vi "Pick&Place_module.vi"() -> ()   [LabVIEW 2016]
uses:
  Classes/Controllers/I-O/Copy of NI-DAQ Folder/NI-DAQ.lvclass
  D:/INTT/V1/Classes/Controllers/I-O/Copy of I-O Folder/I-O.lvclass
  Classes/Controllers/Dispenser/Copy of Ultimus V2 Folder/Ultimus V2.lvclass
  <vilib>/Analysis/coordinate.llb/2D Cartesian Coordinate Rotation (Scalar).vi
  <vilib>/Utility/file.llb/Read Delimited Spreadsheet (DBL).vi
  <vilib>/Utility/file.llb/Write Delimited Spreadsheet (DBL).vi
  Classes/Controllers/Motion/Copy of Motion Folder/Motion.lvclass
  Classes/Controllers/Camera/Copy of Controller Folder/Controller.lvclass
  <vilib>/Analysis/NI_AALPro.lvlib
  Classes/Controllers/I-O/Copy of I-O Folder/I-O.lvclass
panel:
  in  "Ultimus Pressure":i16=20
  in  "Values":bool[](array[boolean])=[FALSE, FALSE]
  out "vacuum on?":bool[](array[boolean])
  out "Array 2":dbl[][](array[numeric])
  out "Measured PickupTool position":dbl[][](array[numeric])
  in  "sampel vacuum":i32[](array[numeric])=[15, 19]
  in  "VacChannel for sample":i32=1
  in  "TrayVaccum":bool
  in  "check height? 2":bool
  in  "check height?":bool
  out "Needle parking position":dbl[](array[numeric])
  out "GlueBox":dbl[][](array[numeric])
  out "appended array":dbl[][](array[numeric])
  in  "chip placement height compensation":dbl=-0.47 format="%#_13g"
  out "Sample on HDI":dbl[][](array[numeric]) format="%#_8g"
  in  "Sensor A/B":bool
  out "Gantry current position":dbl[](array[numeric])
  in  "READ Position":bool
  in  "Needle Height Compenstation\n(glue gap)":dbl=0.34
  in  "Needle Alignment":bool
  in  "Parking position":dbl[](array[numeric])=[625.0, 625.0, 0.0, 0.01]
  in  "GOTO":bool
  in  "Default Pickup Tool Position":dbl[][](array[numeric])=[[153.043, 779.997, 54.962, 0.0365632], [153.043, 779.997, 54.962, 0.0365632]]
  in  "Number of Chips/Sensors \nto be assembled":i32=1
  in  "Default HDI alignment \nmark position":dbl[](array[numeric])=[292.437, 991.477, 79.3487, -0.011805]
  in  "Default HDI size":dbl[](array[numeric])=[24.3371, 231.337, -0.0132064, -0.000194865]
  out "# of tasks excuted":i32
  out "Chips on tray position":dbl[][](array[numeric])
  out "measured HDI size":dbl[](array[numeric])
  in  "Chip tray":dbl[](array[numeric])=[465.031, 710.639, 69.8028, 0.00407755]
  out "Sample position \non HDI":dbl[][](array[numeric])
  in  "Inititalize":bool
  in  "Pick and place":bool
  in  "Deposit Glue":bool
  in  "Measure Pickup Tools":bool
  in  "Measure Samples on tray":bool
  out "default chip and sensor position w.r.t. 1st mark":dbl[][](array[numeric])
  in  "Assembly Type":bool=TRUE
  in  "Stop":bool
  in  "Measure HDI":bool
  out "Measure HDI top-left":dbl[](array[numeric])
  # "Sensor Tray \nVacuum Channel"
  # "Chips"
  # "Sensor 0.3 -> 200 micron glue thickness\nChips 0.34-> 150 micron glue thickness"
  # "Sensors"
  # "Sensor B short"
  # "Sensors B\n(Short)"
  # "Sensors A\n(Long)"
  # "Chips : -0.47-> 60 micron height gap\n               -0.5 -> 90 micron"
  # "Sensor A long"
  # "ACTIONS"
  # "HDI infomation"
  # "chips use channel 0, 2\nsensors use channel 0, 1"
  # "sensor height 69.8471\nchip height 84.693"
  # "Pick and Place"
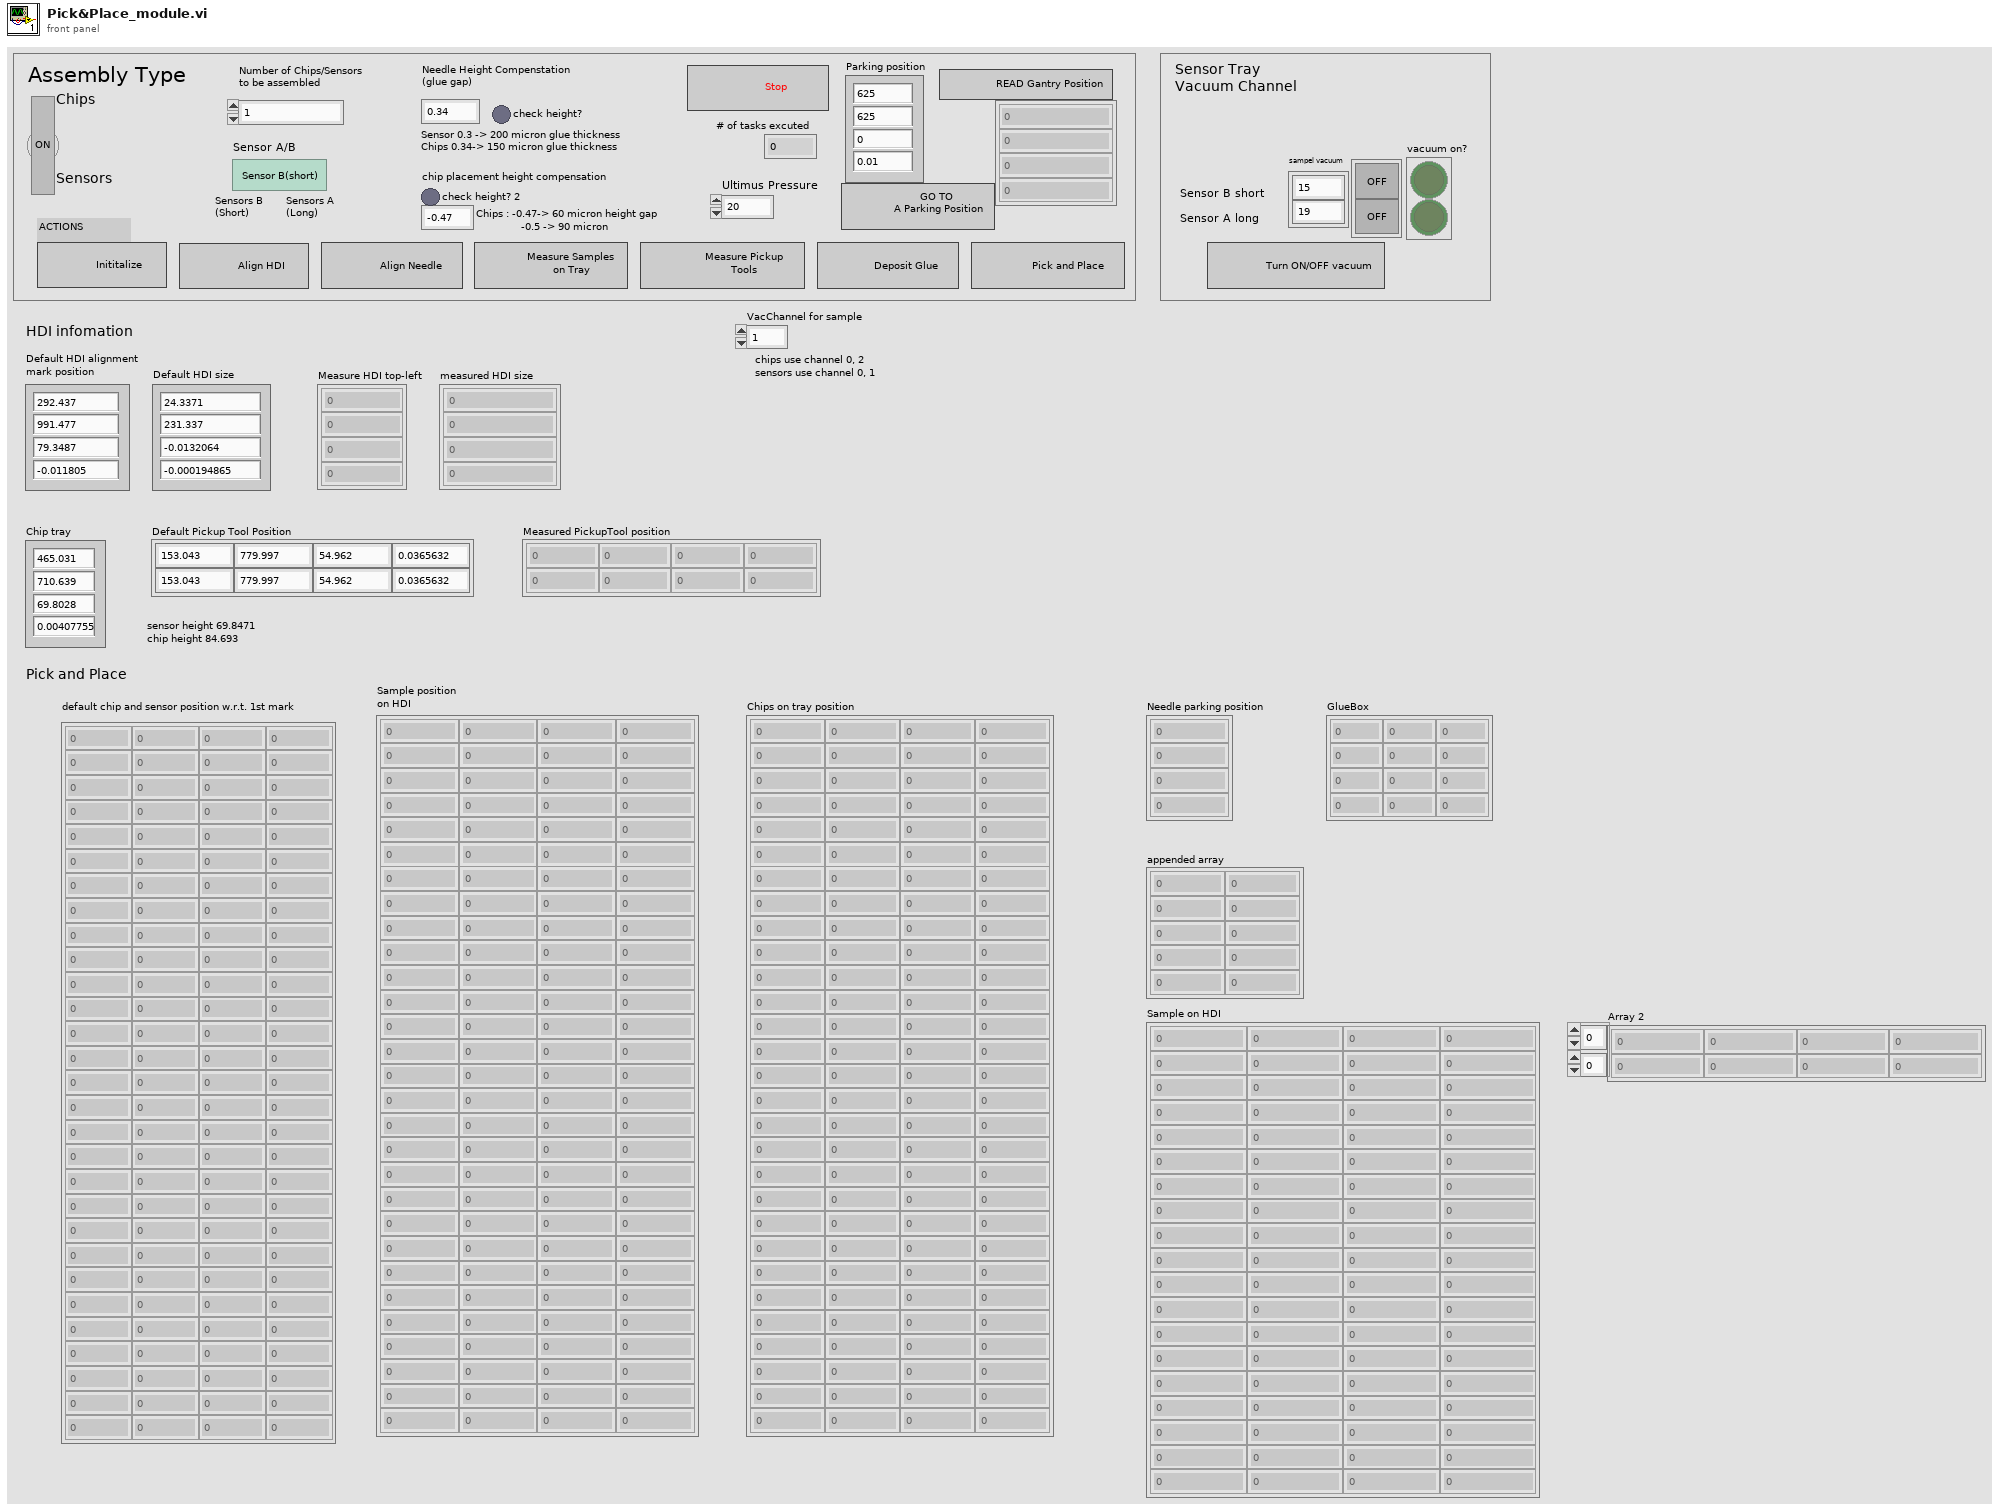
[diagram p1: front panel]
types:
  T1 = typedef "Controller.lvclass/Controllers.ctl" = cluster{"Copy of Motion.lvclass":refnum<class "Motion.lvclass">, "Copy of I-O.lvclass":refnum<class "I-O.lvclass">, "Copy of Dispenser.lvclass":refnum<class "Dispenser.lvclass">}
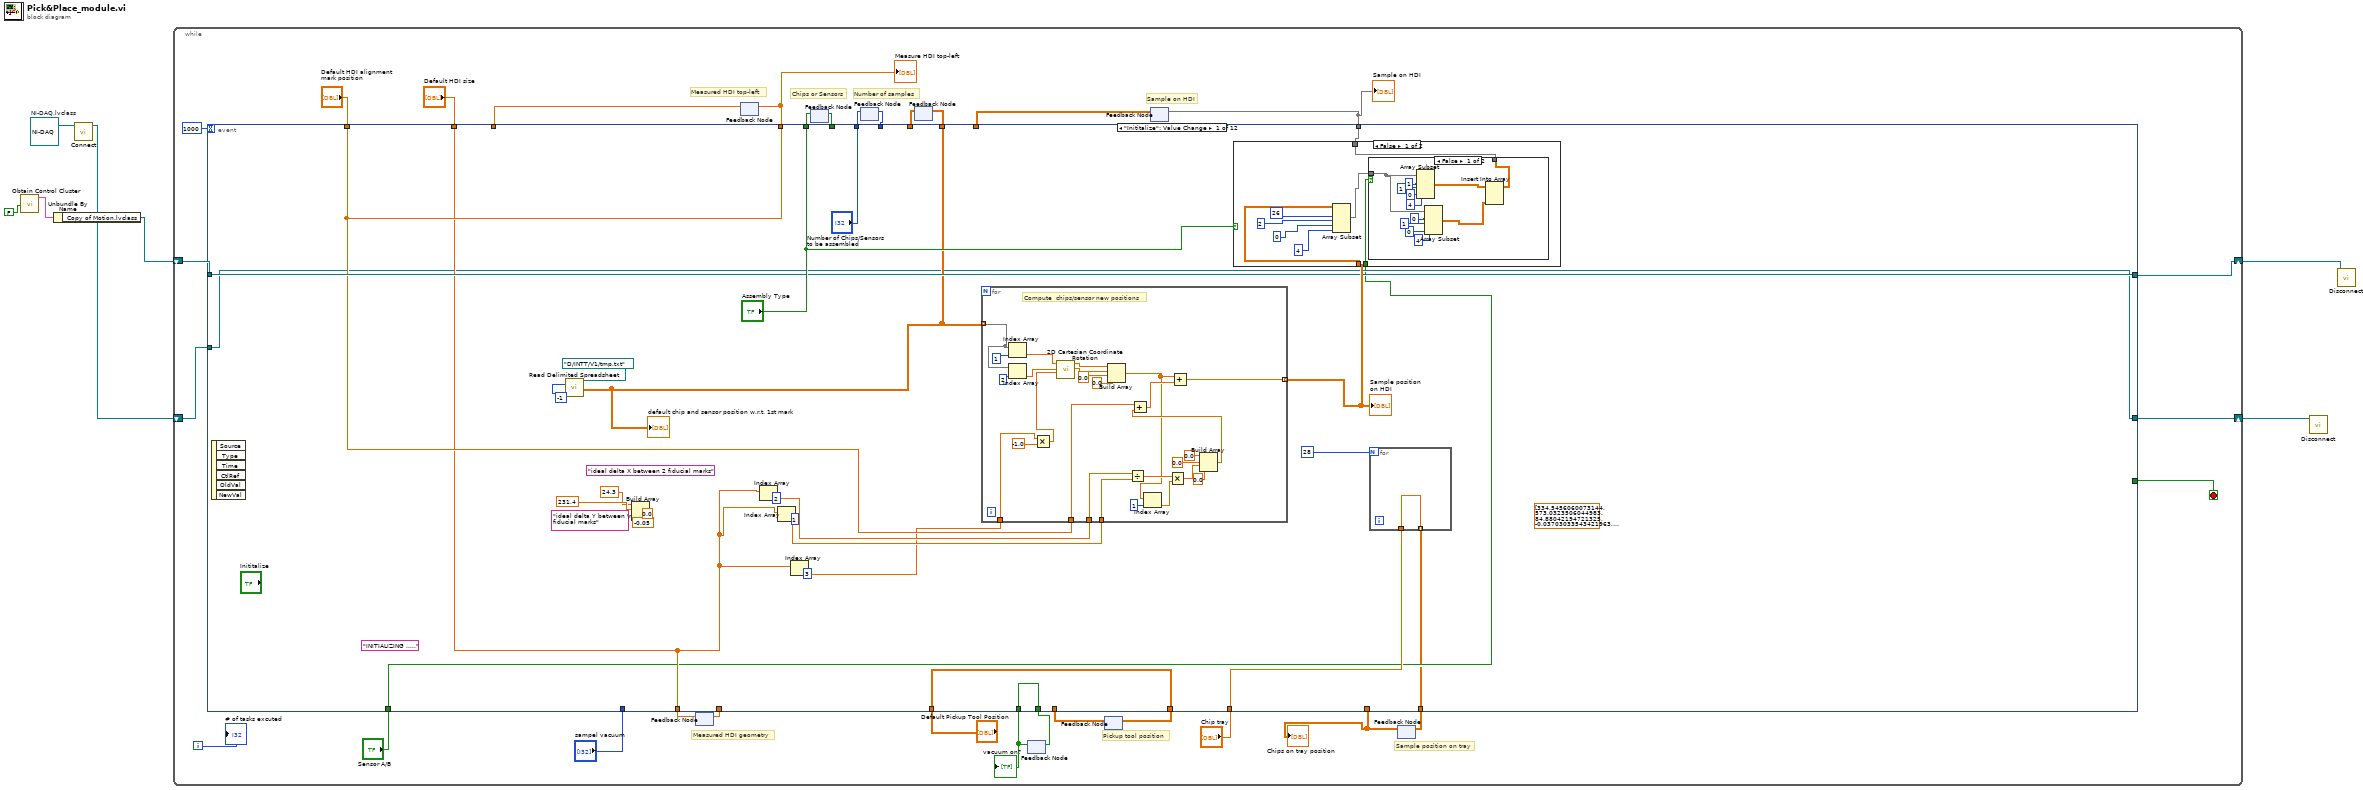
[diagram p0: block diagram]
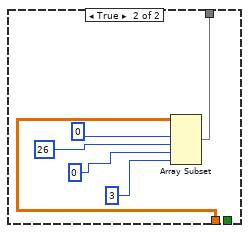
[diagram p3: hidden frame]
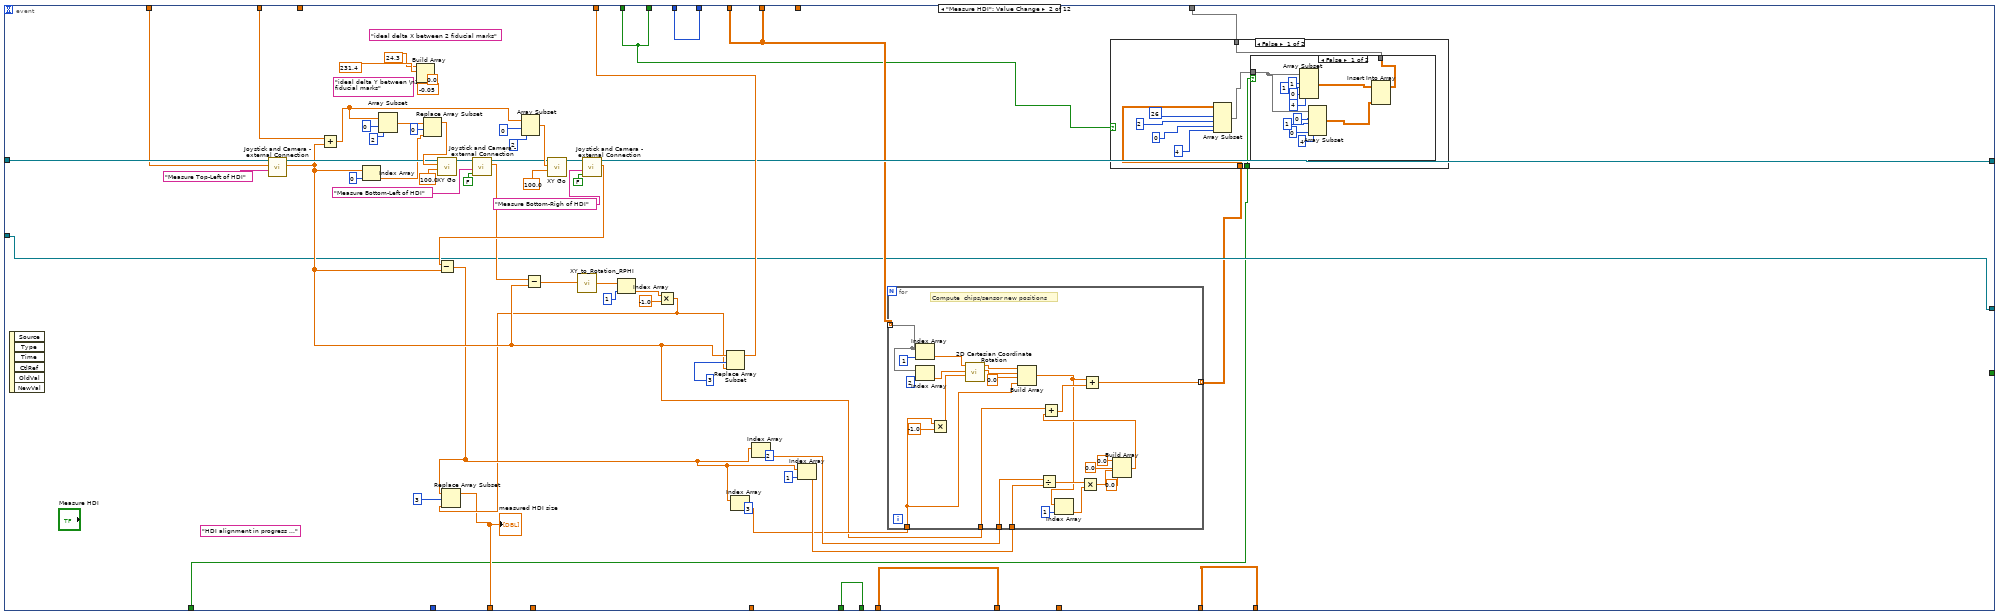
[diagram p4: hidden frame]
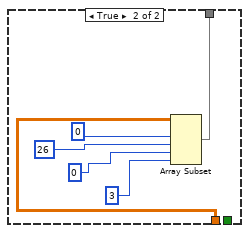
[diagram p6: hidden frame]
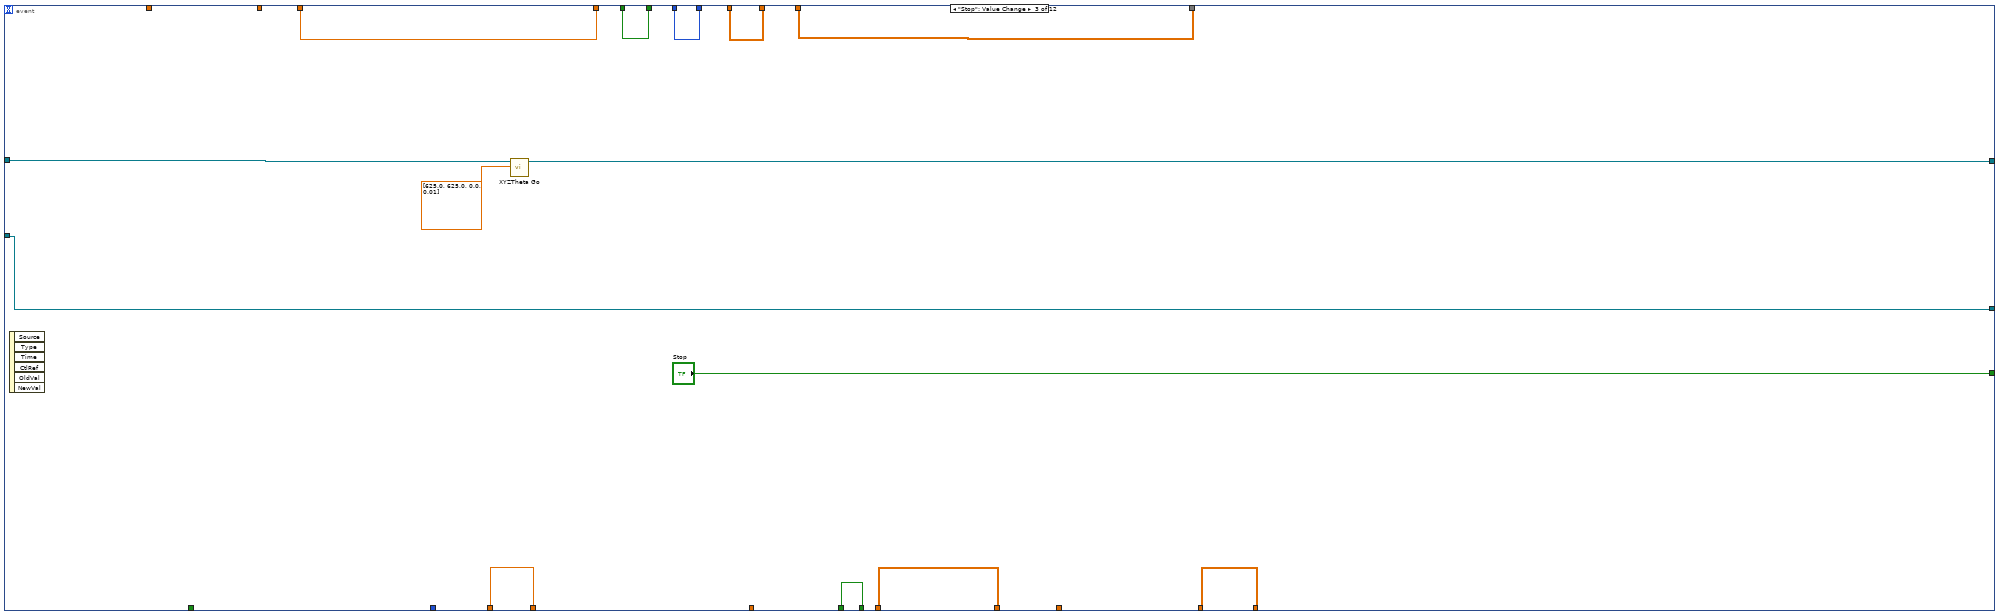
[diagram p7: hidden frame]
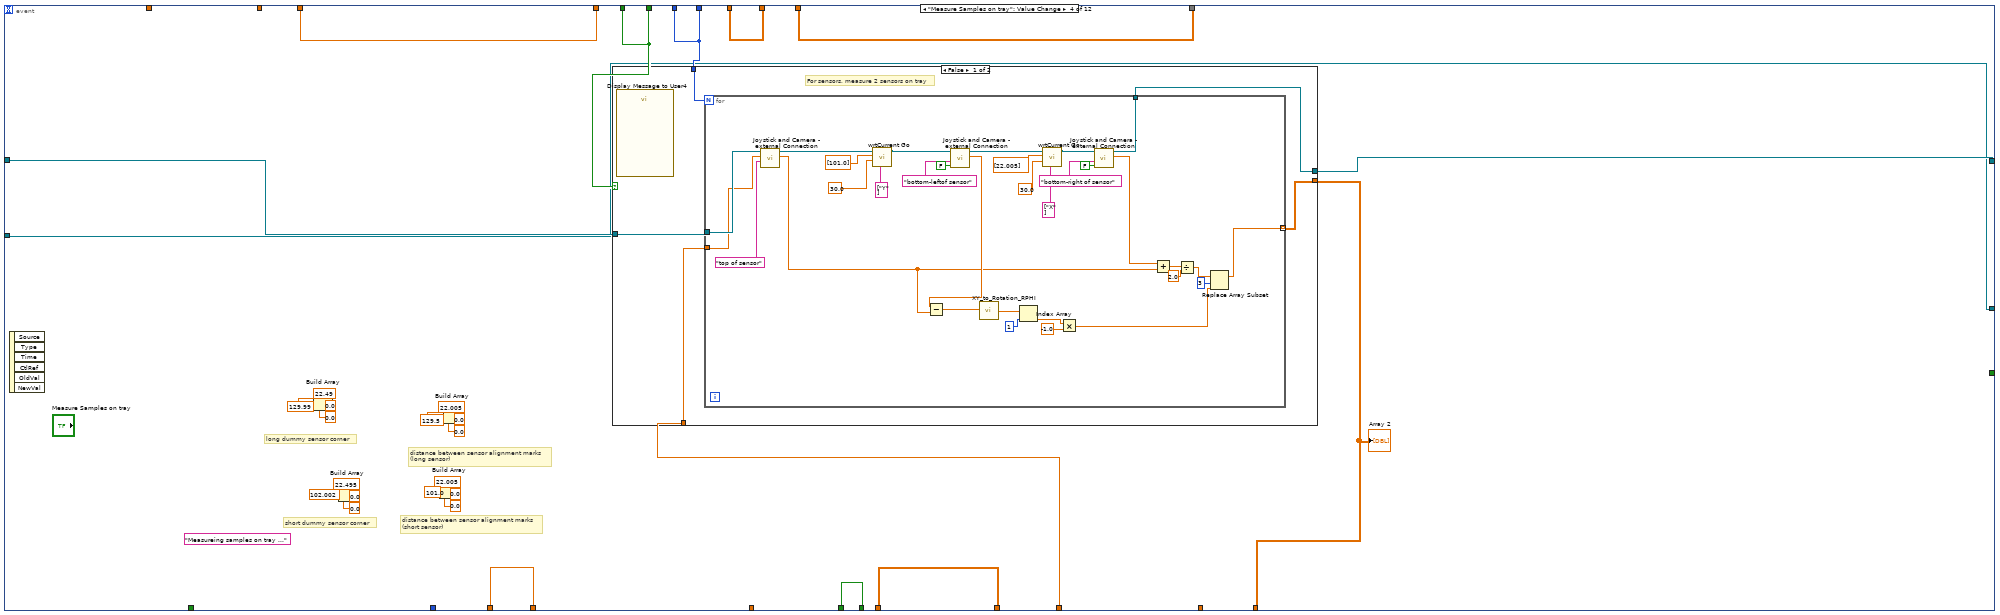
[diagram p8: hidden frame]
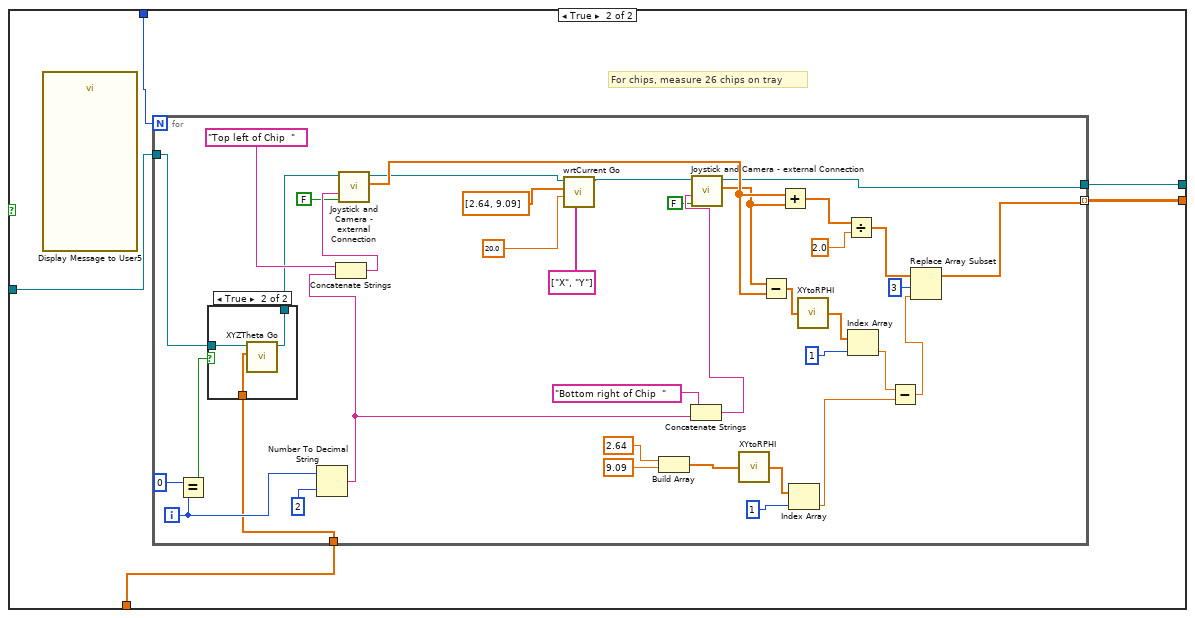
[diagram p9: hidden frame]
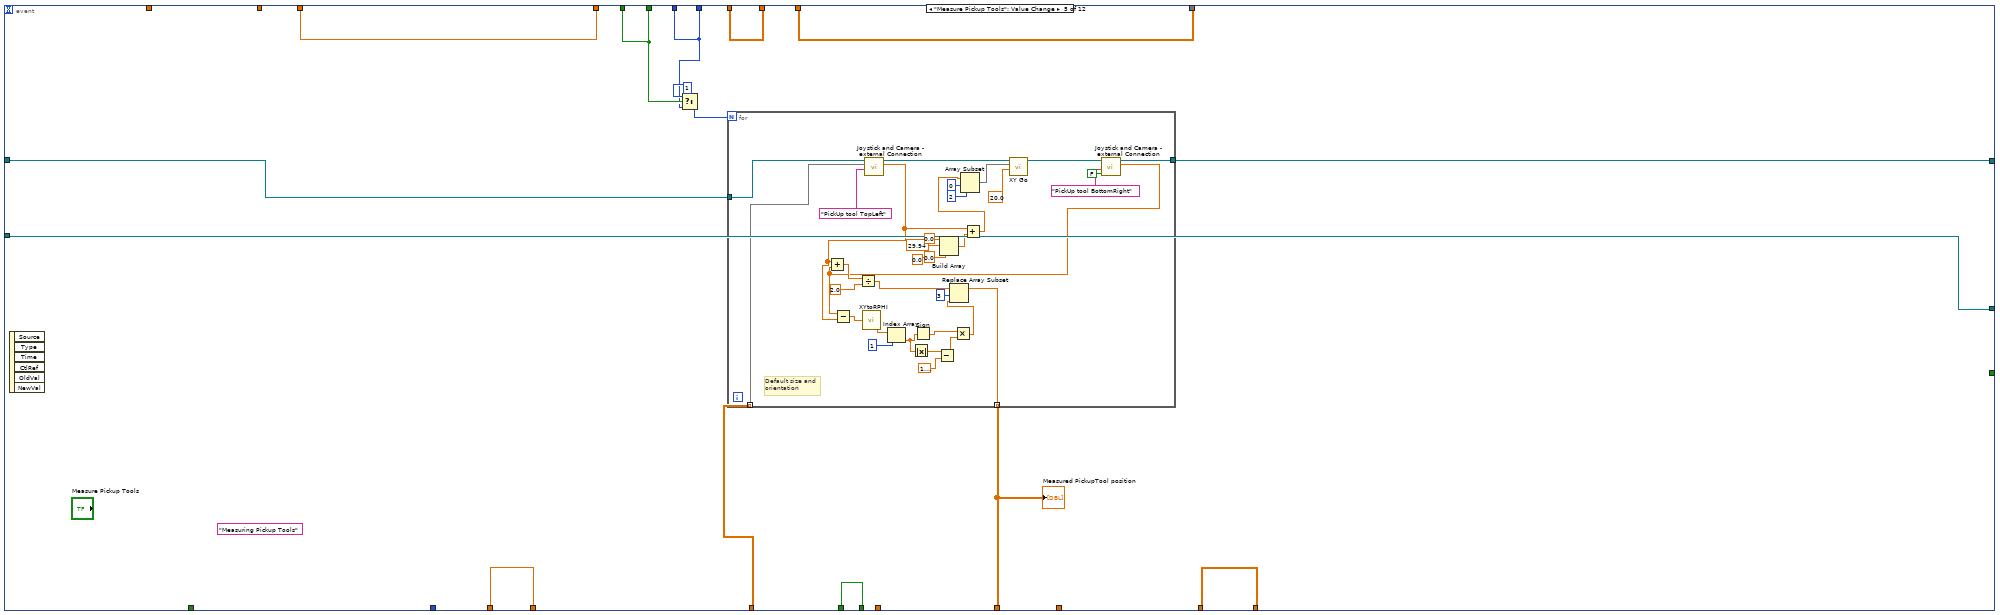
[diagram p11: hidden frame]
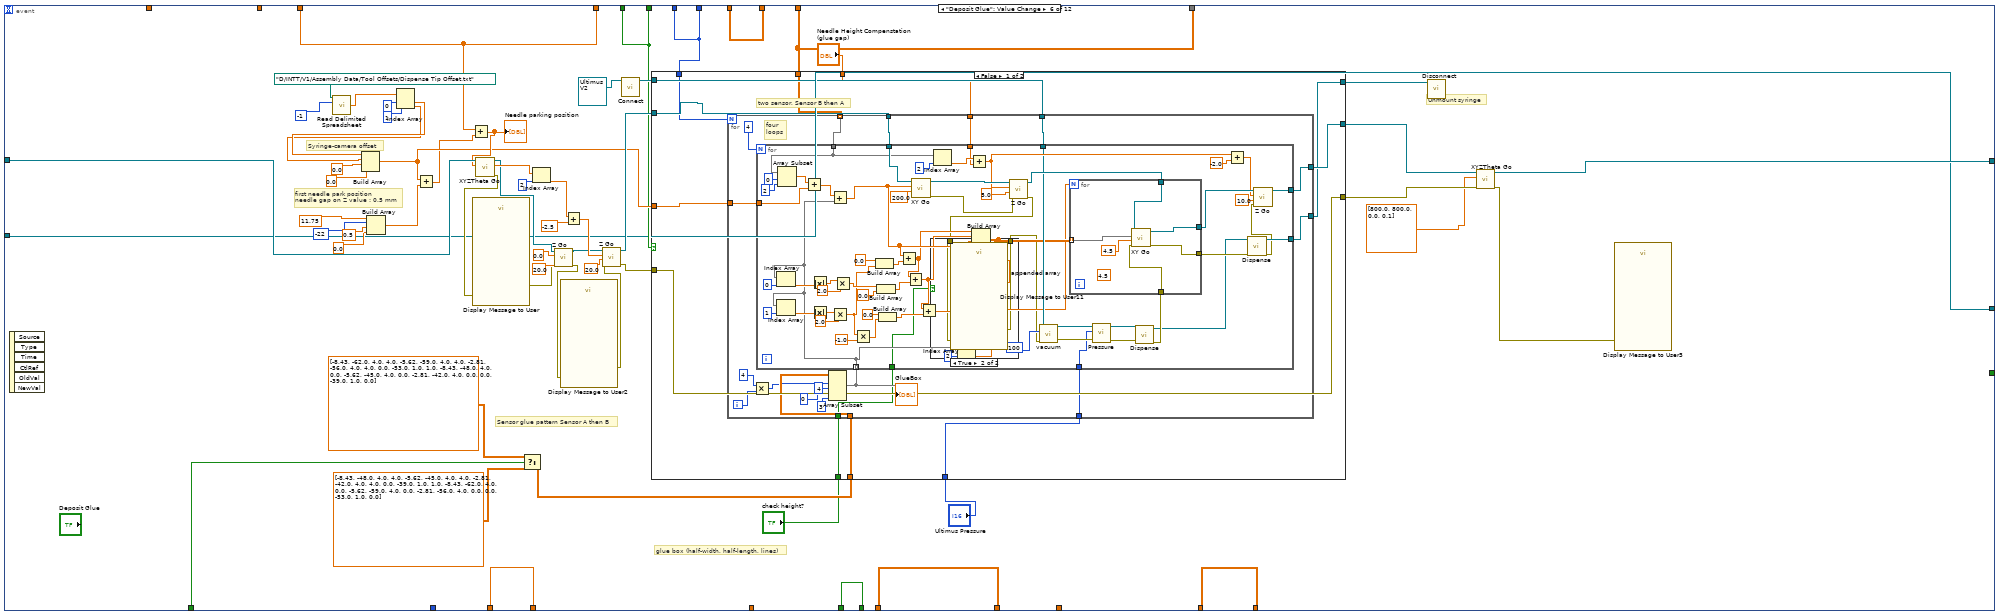
[diagram p12: hidden frame]
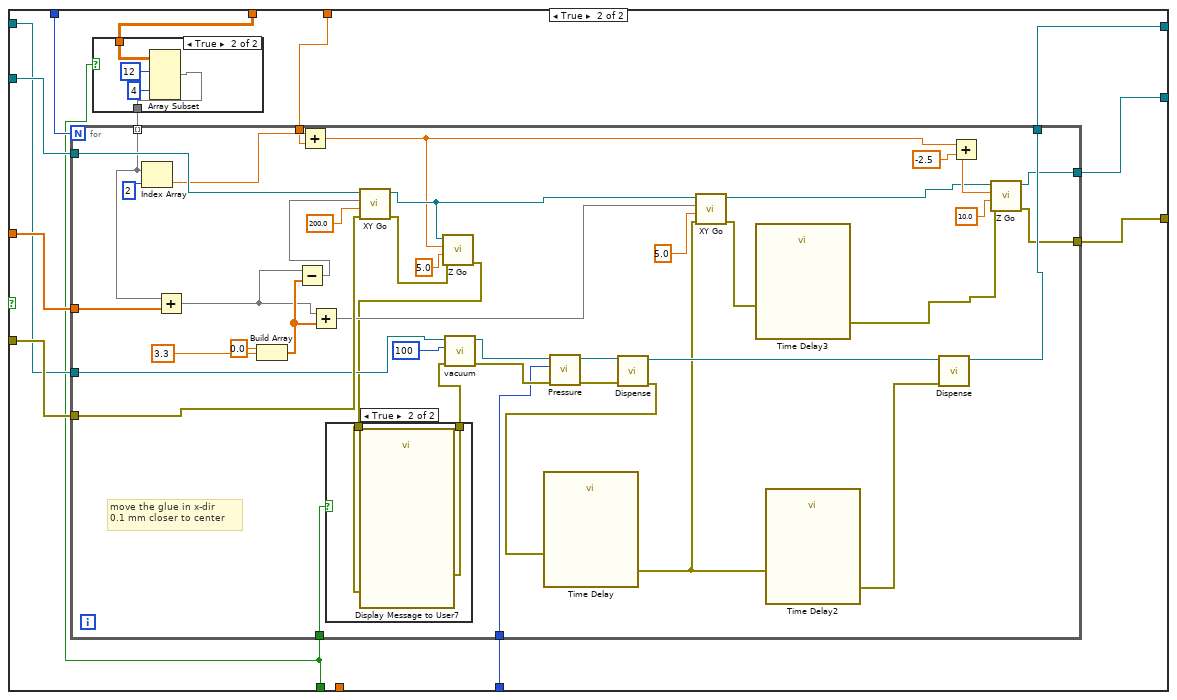
[diagram p14: hidden frame]
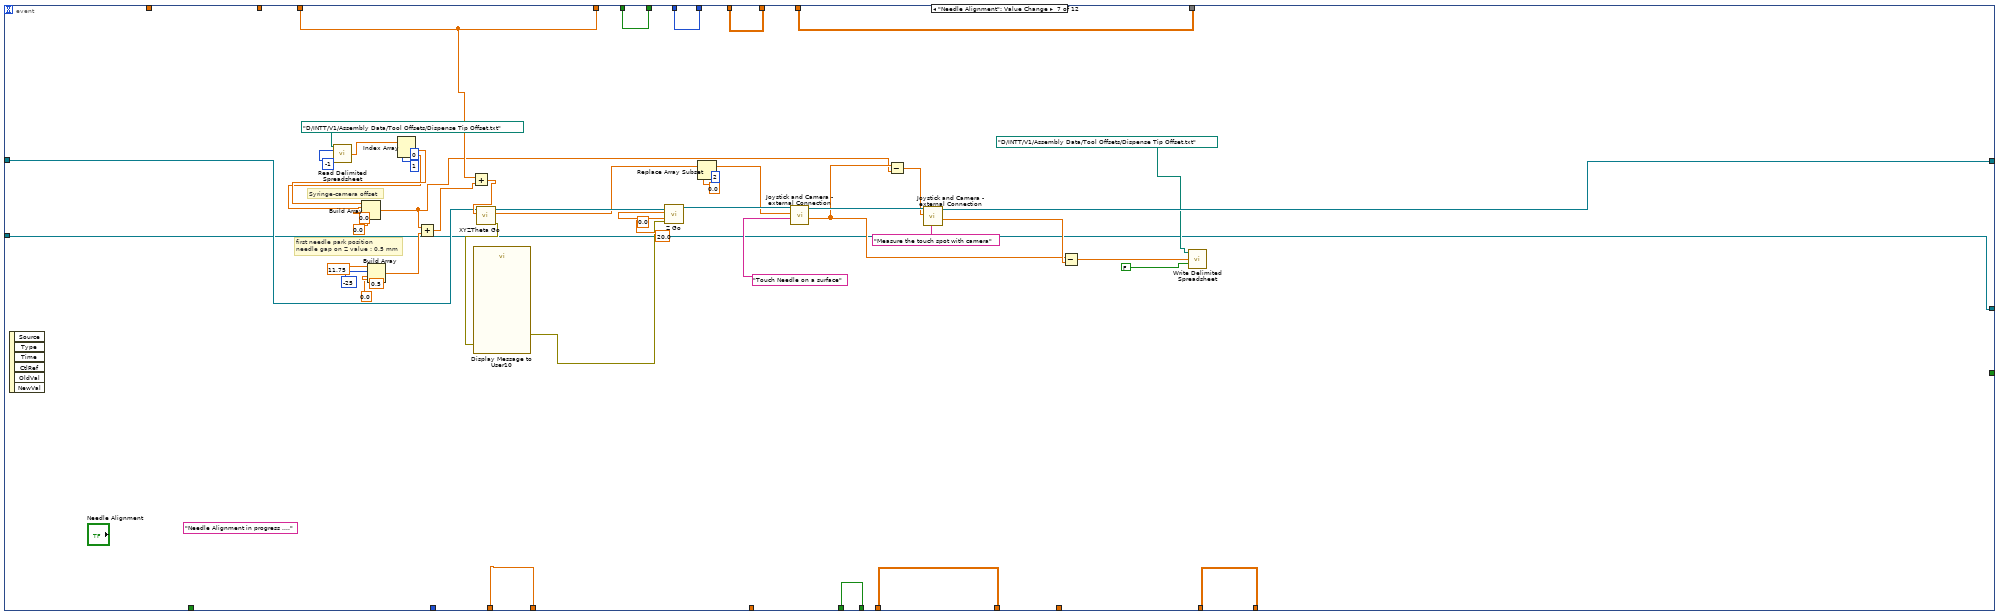
[diagram p17: hidden frame]
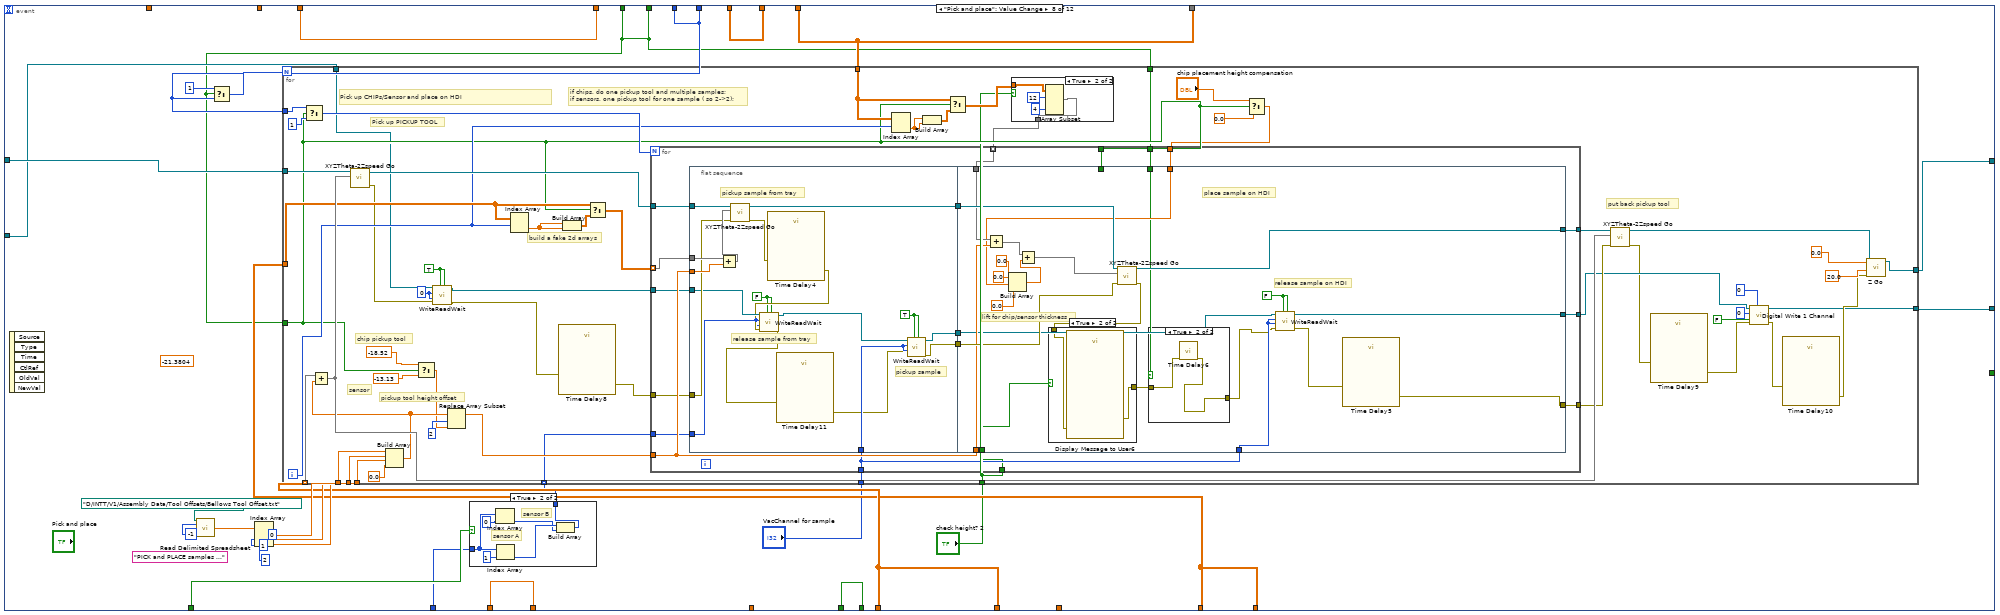
[diagram p18: hidden frame]
diagram:
  w3 = refnum<class "NI-DAQ.lvclass"> refnum  # NI-DAQ.lvclass
  n1 = call "Obtain Control Cluster.vi"("I/O"=FALSE) -> ("Control Out"=w7:T1)  [unwired: 10 in]
  n2 = Unbundle By Name(w7) -> ("Copy of Motion.lvclass"=w5:refnum<class "Motion.lvclass">)
  n3 = call-dynamic "Connect.vi"("NI-DAQ in"=w3) -> ("NI-DAQ out"=w2:refnum<class "NI-DAQ.lvclass">)  [unwired: 9 in, 1 out]
  n4 = while {
    shift-right: [w26] -> w4
    shift-left: w5 -> [w38]
    shift-right: [w12] -> w1
    shift-left: w2 -> [w13]
    i -> [w25]
    stop <- w37 stop-if-true
    # "Pickup tool position"
    # "Chips or Sensors"
    # "Number of samples"
    # "Measured HDI geometry"
    # "Sample position on tray"
    # "Measured HDI top-left"
    # "Sample on HDI"
    n5 = feedback #1() -> (w33:dbl[])  [unwired: 1 in]
    n6 = feedback #2() -> (w35:dbl[])  [unwired: 1 in]
    n7 = feedback #3() -> (w30:bool)  [unwired: 1 in]
    n8 = feedback #4() -> (w24:i32)  [unwired: 1 in]
    n9 = feedback #5() -> (w19:dbl[][])  [unwired: 1 in]
    n10 = feedback #6() -> (w9:bool[])  [unwired: 1 in]
    n11 = feedback #7() -> (w27:dbl[][])  [unwired: 1 in]
    n12 = feedback #8() -> (w32:dbl[][])  [unwired: 1 in]
    n13 = feedback #9() -> (w16:dbl[][])  [unwired: 1 in]
    "Chips on tray position" <- w16
    n14 = event shown="[0] \"Inititalize\": Value Change" {
      selector: _ -> [_ _ _ _ _ _ _ _ _ _ _ _]
      dyn-events: _ -> [_ _ _ _ _ _ _ _ _ _ _ _]
      timeout: 1000 -> [_ _ _ _ _ _ _ _ _ _ _ _]
      tunnel: w38 -> [w52 w179 w245 w274 w372 w441 w649 w705 w846 w868 w892 w894]
      tunnel: [_ _ "Stop" _ _ _ _ _ _ _ _ _] -> w37
      tunnel: [w49 w176 w238 w268 w363 w422 w657 w689 w855 w862 w888 w905] -> w36
      tunnel: w35 -> [_ _ w238 w268 w363 w422 w657 w689 w855 w862 w888 w905]
      tunnel: ["Assembly Type" w122 w242 w272 w368 w425 w656 w679 w854 w863 w889 w904] -> w31
      tunnel: [w45 w126 w237 w267 w362 w418 w652 w688 w850 w861 w887 w898] -> w34
      tunnel: w33 -> [_ _ w237 w267 w362 w418 w652 w688 w850 w861 w887 w898]
      tunnel: [w40 w123 w239 w269 w365 w424 w653 w694 w851 w866 w891 w901] -> w14
      tunnel: w32 -> [_ _ w239 w269 w365 w424 w653 w694 w851 w866 w891 w901]
      tunnel: w30 -> [_ w122 w242 w272 w368 w425 w656 w679 w854 w863 w889 w904]
      tunnel: w24 -> [_ w167 w241 w271 w367 w423 w655 w691 w853 w864 w884 w903]
      tunnel: [w39 w165 w235 w248 w361 w420 w650 w692 w848 w859 w885 w900] -> w29
      tunnel: w16 -> [_ w165 w235 _ w361 w420 w650 w692 w848 w859 w885 w900]
      tunnel: [w48 w166 w236 w266 w371 w419 w651 w693 w849 w860 w886 w899] -> w28
      tunnel: w27 -> [_ w166 w236 w266 _ w419 w651 w693 w849 w860 w886 w899]
      tunnel: [w52 w175 w243 w273 w370 w426 w641 w695 w845 w867 w892 w894] -> w26
      tunnel: ["Number of Chips/Sensors \nto be assembled" w167 w241 w271 w367 w423 w655 w691 w853 w864 w884 w903] -> w23
      tunnel: "Default HDI alignment \nmark position" -> [w49 w174 _ _ _ _ _ _ _ _ _ _]
      tunnel: "Default HDI size" -> [w45 w173 _ _ _ _ _ _ _ _ _ _]
      tunnel: [w50 w168 w240 w270 w364 w417 w654 w690 w852 w865 w890 w902] -> w20
      tunnel: w19 -> [_ w168 w240 w270 w364 w417 w654 w690 w852 w865 w890 w902]
      tunnel: "Default Pickup Tool Position" -> [w48 _ _ _ w366 _ _ _ _ _ _ _]
      tunnel: "Chip tray" -> [w47 _ _ w265 _ _ _ _ _ _ _ _]
      tunnel: "Sensor A/B" -> [w42 w120 _ _ _ w416 _ w687 _ _ _ _]
      tunnel: w13 -> [w43 w125 w233 w247 w360 w410 w632 w684 w847 w857 w883 w895]
      tunnel: [w43 w125 w233 w247 w360 w410 w632 w685 w847 w857 w869 w893] -> w12
      tunnel: "sampel vacuum" -> [_ _ _ _ _ _ _ w681 _ _ w871 w896]
      tunnel: [w41 w124 w232 w246 w359 w409 w631 w680 w843 w856 w870 w897] -> w10
      tunnel: w9 -> [w41 w124 w232 w246 w359 w409 w631 w680 w843 w856 w870 _]
      event "Inititalize": Value Change {
        (unwired) dbl[][] [[334.5456060073144, 573.0323506044983, 84.88042194721325, -0.03703033543421963], [348.7343172517964, 572.8622513715641, 84.88042161151989, 0.002496633181773955], [362.2570314501057, 572.9994237111084, 84.87348419133077, 0.0034316271147138977], [374.6597880882888, 573.1847541366935, 84.85760352984227, -0.00879928913304795], [388.2847032482186, 573.1649677768512, 84.84172357788742, -0.026054726433181852], [334.1328739355822, 593.938164573938, 84.85715223326392, 0.0033385186776999642], [348.32260344605317, 593.1627350557167, 84.85715229429908, 0.032527677556001944], [361.94845426967004, 593.1988990556995, 84.85715231337257, 0.010856722342177383], [375.3711307391728, 592.862734170051, 84.81179255805122, 0.023593691294119035], [388.0023391138823, 592.7263595201845, 84.81179247794259, -0.025867399820654446], [333.741332819156, 613.4501439838673, 84.86893968673877, 0.012458442710573392], [347.4966613938597, 613.1815273693476, 84.84113487130284, 0.02669962172184226], [360.982501589219, 613.368579091193, 84.84113464623572, -0.018470295852746066], [333.329425210144, 634.0016681075332, 84.84113694649815, -0.011509836209115054], [347.60697621578583, 633.6458142671074, 84.84113655739904, -0.014006699863984284], [362.03055194039933, 633.3683242670324, 84.84113543587804, 0.008503358353721735], [374.6669884842355, 633.6776673973038, 84.82931378598124, -0.012163463061963586], [388.449715198344, 634.0661620162508, 84.81749059876144, -0.029966589814424793], [334.6459562288677, 653.6797245247765, 84.85127519810308, -0.010927379491059153], [348.144539580008, 653.7156084768662, 84.88505952278655, -0.012269636914733706], [361.33508542794345, 653.7223221455167, 84.84332432319749, -0.0225512602477429], [374.2287534347454, 653.8981636020831, 84.87276718319089, 0.0007662059738136051], [387.0483029791335, 653.6404602098912, 84.83290343994173, 0.01982829778783901], [334.77129192493265, 669.5351603609607, 84.8979373024785, 0.03923574774306138], [347.17815774254836, 669.4879675513143, 84.9183079020849, 0.003793410140892961], [361.84116966674696, 669.9123563355322, 84.87756716463502, 0.02903318407151878]] ("Chips on tray position")
        (unwired) "INITIALIZING ....." ("String")
        (unwired) "ideal delta Y between \n2 fiducial marks"
        (unwired) "ideal delta X between 2 fiducial marks"
        n15 = event-data() -> ()  [unwired: 1 in, 6 out]
        n16 = call-poly <vilib>:"Read Delimited Spreadsheet.vi"("file path (dialog if empty)"=path "D:/INTT/V1/tmp.txt", "number of rows (all:-1)"=-1) -> ("all rows"=w50:dbl[][])  [unwired: 8 in, 5 out]
        "default chip and sensor position w.r.t. 1st mark" <- w50
        n17 = Build Array(24.3 ("y"), 231.4 ("y"), 0.0 ("element"), -0.05 ("element")) -> ()  [unwired: 1 out]
        n18 = Index Array(array=w45, index=2) -> (element=w61:dbl)
        n19 = Index Array(array=w45, index=1) -> (element=w60:dbl)
        n20 = Index Array(array=w45, index=3) -> (element=w44:dbl)
        n21 = for {
          tunnel: w50 -> [w112] mode=indexing
          tunnel: w44 -> [w95]
          tunnel: w49 -> [w104]
          tunnel: [w111] -> w54 mode=indexing
          tunnel: w61 -> [w110]
          tunnel: w60 -> [w101]
          # "Compute  chips/sensor new positions"
          n22 = Index Array(array=w112, index=1) -> (element=w116:dbl)
          n23 = Index Array(array=w112, index=2) -> (element=w115:dbl)
          n24 = Multiply(x=w95, y=-1.0) -> (x*y=w96:dbl)
          n25 = call-poly <vilib>:"2D Cartesian Coordinate Rotation.vi"("theta"=w96, "y"=w115, "x"=w116) -> ("y out"=w118:dbl, "x out"=w117:dbl)  [unwired: 6 in, 1 out]
          n26 = Build Array(w117, w118, 0.0 ("element"), 0.0 ("element")) -> (w98:dbl[])
          n27 = Divide(x=w110, y=w101) -> (x/y=w109:dbl)
          n28 = Index Array(array=w98, index=1) -> (element=w99:dbl)
          n29 = Multiply(x=w109, y=w99) -> (x*y=w105:dbl)
          n30 = Build Array(0.0 ("element"), 0.0 ("element"), w105, 0.0 ("element")) -> (w103:dbl[])
          n31 = Add(x=w104, y=w103) -> (x+y=w102:dbl[])
          n32 = Add(x=w98, y=w102) -> (x+y=w111:dbl[])
        }
        "Sample position \non HDI" <- w54
        n33 = case shown="False" "Assembly Type" {
          tunnel: w54 -> [w69 w89]
          tunnel: [w67 w87] -> w40
          tunnel: w42 -> [w66 _]
          frame False {
            n34 = Array Subset(array=w69, index (row)=26 ("index"), length (row)=2 ("length"), index (col)=0, length (col)=4 ("length")) -> (w68:dbl[][])
            n35 = case shown="False" w66 {
              tunnel: w68 -> [w77 w86]
              tunnel: [w74 w86] -> w67
              frame False {
                n36 = Array Subset(array=w77, index (row)=1 ("index"), length (row)=1 ("length"), index (col)=0 ("index"), length (col)=4 ("length")) -> (w76:dbl[][])
                n37 = Array Subset(array=w77, index (row)=0 ("index"), length (row)=1 ("length"), index (col)=0 ("index"), length (col)=4 ("length")) -> (w75:dbl[][])
                n38 = Insert Into Array(array=w76, new element=w75) -> (w74:dbl[][])  [unwired: 2 in]
              }
              frame True {
              }
            }
          }
          frame True {
            n39 = Array Subset(array=w89, index (row)=0 ("index"), length (row)=26 ("length"), index (col)=0, length (col)=3 ("length")) -> (w87:dbl[][])
          }
        }
        n40 = for {
          N: 28 -> [_]
          tunnel: w47 -> [w93]
          tunnel: [w93] -> w39 mode=indexing
        }
      }
      event "Measure HDI": Value Change {
        (unwired) "ideal delta Y between \n2 fiducial marks"
        (unwired) "ideal delta X between 2 fiducial marks"
        (unwired) "HDI alignment in progress ..." ("String")
        n41 = event-data() -> ()  [unwired: 1 in, 6 out]
        n42 = call "Joystick and Camera - external Connection.vi"("Motion in"=w179, "XYZTheta"=w174, "Measurement Point"="Measure Top-Left of HDI") -> ("Motion out"=w143:refnum<class "Motion.lvclass">, "Sum"=w132:dbl[])  [unwired: 4 in, 2 out]
        n43 = Add(x=w173, y=w132) -> (x+y=w147:dbl[])
        n44 = Index Array(array=w132, index=0) -> (element=w134:dbl)
        n45 = Array Subset(array=w147, index=0, length=2) -> (w146:dbl[])
        n46 = Build Array(24.3 ("y"), 231.4 ("y"), 0.0 ("element"), -0.05 ("element")) -> ()  [unwired: 1 out]
        n47 = Replace Array Subset(array=w146, new element=w134, index=0) -> (w144:dbl[])
        n48 = call-dynamic "XY Go.vi"("Speed"=100.0, "XY"=w144, "Motion in"=w143) -> ("Motion out"=w151:refnum<class "Motion.lvclass">)  [unwired: 7 in, 1 out]
        n49 = call "Joystick and Camera - external Connection.vi"("Motion in"=w151, "Measurement Point"="Measure Bottom-Left of HDI", "Inital GO"=FALSE) -> ("Motion out"=w142:refnum<class "Motion.lvclass">, "Sum"=w133:dbl[])  [unwired: 4 in, 2 out]
        n50 = Array Subset(array=w147, index=0, length=2) -> (w157:dbl[])
        n51 = Subtract(x=w133, y=w132) -> (x-y=w141:dbl[])
        n52 = call-dynamic "XY Go.vi"("Speed"=100.0, "XY"=w157, "Motion in"=w142) -> ("Motion out"=w161:refnum<class "Motion.lvclass">)  [unwired: 7 in, 1 out]
        n53 = call "XY_to_Rotation_RPHI.vi"("X-Y"=w141) -> ("r-phi"=w137:dbl[])
        n54 = call "Joystick and Camera - external Connection.vi"("Motion in"=w161, "Measurement Point"="Measure Bottom-Righ of HDI", "Inital GO"=FALSE) -> ("Motion out"=w175:refnum<class "Motion.lvclass">, "Sum"=w178:dbl[])  [unwired: 4 in, 2 out]
        n55 = Subtract(x=w178, y=w132) -> (x-y=w129:dbl[])
        n56 = Index Array(array=w137, index=1) -> (element=w130:dbl)
        n57 = Multiply(x=w130, y=-1.0) -> (x*y=w127:dbl)
        n58 = Replace Array Subset(array=w129, new element=w127, index=3) -> (w126:dbl[])
        "measured HDI size" <- w126
        n59 = Replace Array Subset(array=w132, new element=w127, index=3) -> (w176:dbl[])
        n60 = Index Array(array=w129, index=3) -> (element=w163:dbl)
        n61 = Index Array(array=w129, index=2) -> (element=w170:dbl)
        n62 = Index Array(array=w129, index=1) -> (element=w169:dbl)
        n63 = for {
          tunnel: w168 -> [w224] mode=indexing
          tunnel: w163 -> [w208]
          tunnel: w132 -> [w216]
          tunnel: [w223] -> w121 mode=indexing
          tunnel: w170 -> [w222]
          tunnel: w169 -> [w213]
          # "Compute  chips/sensor new positions"
          n64 = Index Array(array=w224, index=1) -> (element=w228:dbl)
          n65 = Index Array(array=w224, index=2) -> (element=w227:dbl)
          n66 = Multiply(x=w208, y=-1.0) -> (x*y=w207:dbl)
          n67 = call-poly <vilib>:"2D Cartesian Coordinate Rotation.vi"("theta"=w207, "y"=w227, "x"=w228) -> ("y out"=w230:dbl, "x out"=w229:dbl)  [unwired: 6 in, 1 out]
          n68 = Build Array(w229, w230, 0.0 ("element"), w208) -> (w210:dbl[])
          n69 = Divide(x=w222, y=w213) -> (x/y=w221:dbl)
          n70 = Index Array(array=w210, index=1) -> (element=w211:dbl)
          n71 = Multiply(x=w221, y=w211) -> (x*y=w217:dbl)
          n72 = Build Array(0.0 ("element"), 0.0 ("element"), w217, 0.0 ("element")) -> (w215:dbl[])
          n73 = Add(x=w216, y=w215) -> (x+y=w214:dbl[])
          n74 = Add(x=w210, y=w214) -> (x+y=w223:dbl[])
        }
        n75 = case shown="False" w122 {
          tunnel: w121 -> [w183 w203]
          tunnel: [w181 w201] -> w123
          tunnel: w120 -> [w180 _]
          frame False {
            n76 = Array Subset(array=w183, index (row)=26 ("index"), length (row)=2 ("length"), index (col)=0, length (col)=4 ("length")) -> (w182:dbl[][])
            n77 = case shown="False" w180 {
              tunnel: w182 -> [w191 w200]
              tunnel: [w188 w200] -> w181
              frame False {
                n78 = Array Subset(array=w191, index (row)=1 ("index"), length (row)=1 ("length"), index (col)=0 ("index"), length (col)=4 ("length")) -> (w190:dbl[][])
                n79 = Array Subset(array=w191, index (row)=0 ("index"), length (row)=1 ("length"), index (col)=0 ("index"), length (col)=4 ("length")) -> (w189:dbl[][])
                n80 = Insert Into Array(array=w190, new element=w189) -> (w188:dbl[][])  [unwired: 2 in]
              }
              frame True {
              }
            }
          }
          frame True {
            n81 = Array Subset(array=w203, index (row)=0 ("index"), length (row)=26 ("length"), index (col)=0, length (col)=3 ("length")) -> (w201:dbl[][])
          }
        }
      }
      event "Stop": Value Change {
        n82 = event-data() -> ()  [unwired: 1 in, 6 out]
        n83 = call "XYZTheta Go.vi"("XYZTheta In"=dbl[] [625.0, 625.0, 0.0, 0.01], "Motion in"=w245) -> ("Motion out"=w243:refnum<class "Motion.lvclass">)  [unwired: 7 in, 2 out]
      }
      event "Measure Samples on tray": Value Change {
        (unwired) "Measureing samples on tray ..." ("String")
        # "long dummy sensor corner"
        # "short dummy sensor corner"
        # "distance between sensor alignment marks\n(short sensor)"
        # "distance between sensor alignment marks\n(long sensor)"
        n84 = event-data() -> ()  [unwired: 1 in, 6 out]
        n85 = Build Array(22.49 ("element"), 129.99 ("element"), 0.0 ("element"), 0.0 ("element")) -> ()  [unwired: 1 out]
        n86 = Build Array(22.495 ("element"), 102.002 ("element"), 0.0 ("element"), 0.0 ("element")) -> ()  [unwired: 1 out]
        n87 = Build Array(22.005 ("element"), 101.0 ("element"), 0.0 ("element"), 0.0 ("element")) -> ()  [unwired: 1 out]
        n88 = Build Array(22.005 ("element"), 129.5 ("element"), 0.0 ("element"), 0.0 ("element")) -> ()  [unwired: 1 out]
        n89 = case shown="False" w272 {
          tunnel: [w276 w316] -> w248
          tunnel: w274 -> [w279 w315]
          tunnel: [w275 w314] -> w273
          tunnel: w271 -> [w278 w313]
          tunnel: w265 -> [w277 w312]
          frame False {
            # "For sensors, measure 2 sensors on tray"
            n90 = call "Display Message to User4"() -> ()  [unwired: 10 in, 2 out]
            n91 = for {
              N: w278 -> [_]
              tunnel: w279 -> [w311]
              tunnel: [w308] -> w275
              tunnel: [w302] -> w276 mode=indexing
              tunnel: w277 -> [w301]
              n92 = call "Joystick and Camera - external Connection.vi"("Motion in"=w311, "XYZTheta"=w301, "Measurement Point"="top of sensor") -> ("Motion out"=w283:refnum<class "Motion.lvclass">, "Sum"=w290:dbl[])  [unwired: 4 in, 2 out]
              n93 = call-dynamic "wrtCurrent Go.vi"("axis names"=string[] ["Y"], "Speed"=30.0, "distances"=dbl[] [101.0], "Motion in"=w283) -> ("Motion out"=w282:refnum<class "Motion.lvclass">)  [unwired: 6 in, 1 out]
              n94 = call "Joystick and Camera - external Connection.vi"("Motion in"=w282, "Measurement Point"="bottom-leftof sensor", "Inital GO"=FALSE) -> ("Motion out"=w288:refnum<class "Motion.lvclass">, "Sum"=w292:dbl[])  [unwired: 4 in, 2 out]
              n95 = Subtract(x=w292, y=w290) -> (x-y=w297:dbl[])
              n96 = call "XY_to_Rotation_RPHI.vi"("X-Y"=w297) -> ("r-phi"=w296:dbl[])
              n97 = Index Array(array=w296, index=1) -> (element=w293:dbl)
              n98 = call-dynamic "wrtCurrent Go.vi"("axis names"=string[] ["X"], "Speed"=30.0, "distances"=dbl[] [22.005], "Motion in"=w288) -> ("Motion out"=w289:refnum<class "Motion.lvclass">)  [unwired: 6 in, 1 out]
              n99 = Multiply(x=w293, y=-1.0) -> (x*y=w291:dbl)
              n100 = call "Joystick and Camera - external Connection.vi"("Motion in"=w289, "Measurement Point"="bottom-right of sensor", "Inital GO"=FALSE) -> ("Motion out"=w308:refnum<class "Motion.lvclass">, "Sum"=w305:dbl[])  [unwired: 4 in, 2 out]
              n101 = Add(x=w305, y=w290) -> (x+y=w306:dbl[])
              n102 = Divide(x=w306, y=2.0) -> (x/y=w304:dbl[])
              n103 = Replace Array Subset(array=w304, new element=w291, index=3) -> (w302:dbl[])
            }
          }
          frame True {
            # "For chips, measure 26 chips on tray"
            n104 = call "Display Message to User5"() -> ()  [unwired: 10 in, 2 out]
            n105 = for {
              N: w313 -> [_]
              tunnel: [w343] -> w316 mode=indexing
              tunnel: w315 -> [w327]
              tunnel: [w323] -> w314
              tunnel: w312 -> [w328]
              i -> [w331]
              n106 = Equal?(x=0, y=w331) -> (x = y?=w329:bool)
              n107 = case shown="True" w329 {
                tunnel: w328 -> [_ w358]
                tunnel: w327 -> [w355 w357]
                tunnel: [w355 w356] -> w326
                frame False {
                }
                frame True {
                  n108 = call "XYZTheta Go.vi"("XYZTheta In"=w358, "Motion in"=w357) -> ("Motion out"=w356:refnum<class "Motion.lvclass">)  [unwired: 7 in, 2 out]
                }
              }
              n109 = Number To Decimal String(number=w331, width (-)=i16 2) -> (decimal integer string=w347:string)
              n110 = Concatenate Strings("Top left of Chip  " ("string"), w347) -> (w341:string)
              n111 = call "Joystick and Camera - external Connection.vi"("Motion in"=w326, "Measurement Point"=w341, "Inital GO"=FALSE) -> ("Motion out"=w320:refnum<class "Motion.lvclass">, "Sum"=w346:dbl[])  [unwired: 4 in, 2 out]
              n112 = call-dynamic "wrtCurrent Go.vi"("axis names"=string[] ["X", "Y"], "Speed"=20.0, "distances"=dbl[] [2.64, 9.09], "Motion in"=w320) -> ("Motion out"=w321:refnum<class "Motion.lvclass">)  [unwired: 6 in, 1 out]
              n113 = Build Array(2.64 ("element"), 9.09 ("element")) -> (w336:dbl[])
              n114 = Concatenate Strings("Bottom right of Chip  " ("string"), w347) -> (w325:string)
              n115 = call "Joystick and Camera - external Connection.vi"("Motion in"=w321, "Measurement Point"=w325, "Inital GO"=FALSE) -> ("Motion out"=w323:refnum<class "Motion.lvclass">, "Sum"=w322:dbl[])  [unwired: 4 in, 2 out]
              n116 = call "XYtoRPHI.vi"("X-Y"=w336) -> ("r-phi"=w338:dbl[])
              n117 = Subtract(x=w322, y=w346) -> (x-y=w339:dbl[])
              n118 = Add(x=w346, y=w322) -> (x+y=w351:dbl[])
              n119 = Index Array(array=w338, index=1) -> (element=w333:dbl)
              n120 = call "XYtoRPHI.vi"("X-Y"=w339) -> ("r-phi"=w350:dbl[])
              n121 = Divide(x=w351, y=2.0) -> (x/y=w345:dbl[])
              n122 = Index Array(array=w350, index=1) -> (element=w334:dbl)
              n123 = Subtract(x=w334, y=w333) -> (x-y=w335:dbl)
              n124 = Replace Array Subset(array=w345, new element=w335, index=3) -> (w343:dbl[])
            }
          }
        }
        "Array 2" <- w248
      }
      event "Measure Pickup Tools": Value Change {
        (unwired) "Measuring Pickup Tools" ("String")
        n125 = event-data() -> ()  [unwired: 1 in, 6 out]
        n126 = Select(t=i8 1, s=w368, f=w367) -> (s? t:f=w369:i32)
        n127 = for {
          N: w369 -> [_]
          tunnel: [w397] -> w371 mode=indexing
          tunnel: w372 -> [w401]
          tunnel: [w383] -> w370
          tunnel: w366 -> [w382] mode=indexing
          # "Default size and\norientation"
          n128 = call "Joystick and Camera - external Connection.vi"("Motion in"=w401, "XYZTheta"=w382, "Measurement Point"="PickUp tool TopLeft") -> ("Motion out"=w377:refnum<class "Motion.lvclass">, "Sum"=w400:dbl[])  [unwired: 4 in, 2 out]
          n129 = Build Array(0.0 ("element"), 29.94 ("element"), 0.0 ("element"), 0.0 ("element")) -> (w388:dbl[])
          n130 = Add(x=w400, y=w388) -> (x+y=w374:dbl[])
          n131 = Array Subset(array=w374, index=0, length=2) -> (w375:dbl[])
          n132 = call-dynamic "XY Go.vi"("Speed"=20.0, "XY"=w375, "Motion in"=w377) -> ("Motion out"=w376:refnum<class "Motion.lvclass">)  [unwired: 7 in, 1 out]
          n133 = call "Joystick and Camera - external Connection.vi"("Motion in"=w376, "Measurement Point"="PickUp tool BottomRight", "Inital GO"=FALSE) -> ("Motion out"=w383:refnum<class "Motion.lvclass">, "Sum"=w399:dbl[])  [unwired: 4 in, 2 out]
          n134 = Add(x=w400, y=w399) -> (x+y=w406:dbl[])
          n135 = Subtract(x=w399, y=w400) -> (x-y=w398:dbl[])
          n136 = Divide(x=w406, y=2.0) -> (x/y=w403:dbl[])
          n137 = call "XYtoRPHI.vi"("X-Y"=w398) -> ("r-phi"=w404:dbl[])
          n138 = Index Array(array=w404, index=1) -> (element=w392:dbl)
          n139 = Absolute Value(x=w392) -> (abs(x)=w395:dbl)
          n140 = Sign(1:w392) -> (0:w393:dbl)
          n141 = Subtract(x=w395, y=1.5707963267948966) -> (x-y=w394:dbl)
          n142 = Multiply(x=w393, y=w394) -> (x*y=w391:dbl)
          n143 = Replace Array Subset(array=w403, new element=w391, index=3) -> (w397:dbl[])
        }
        "Measured PickupTool position" <- w371
      }
      event "Deposit Glue": Value Change {
        # "glue box (half-width, half-length, lines)"
        # "Sensor glue pattern Sensor A then B"
        # "Unmount syringe"
        # "first needle park position\nneedle gap on Z value : 0.5 mm"
        # "Syringe-camera offset"
        n144 = event-data() -> ()  [unwired: 1 in, 6 out]
        n145 = call-poly <vilib>:"Read Delimited Spreadsheet.vi"("file path (dialog if empty)"=path "D:/INTT/V1/Assembly Data/Tool Offsets/Dispense Tip Offset.txt", "number of rows (all:-1)"=-1) -> ("first row"=w461:dbl[])  [unwired: 8 in, 5 out]
        n146 = Build Array(11.75, -22, 0.5 ("element"), 0.0 ("element")) -> (w454:dbl[])
        n147 = Index Array(array=w461, index #1=0 ("index"), index #2=1 ("index")) -> (element #1=w456:dbl, element #2=w453:dbl)
        n148 = Build Array(w456, w453, 0.0 ("element"), 0.0 ("element")) -> (w434:dbl[])
        n149 = Add(x=w434, y=w454) -> (x+y=w421:dbl[])
        n150 = Add(x=w422, y=w421) -> (x+y=w440:dbl[])
        "Needle parking position" <- w440
        n151 = call "XYZTheta Go.vi"("XYZTheta In"=w440, "Motion in"=w441) -> ("error out"=w452:errorcluster, "XYZTheta Out"=w450:dbl[], "Motion out"=w439:refnum<class "Motion.lvclass">)  [unwired: 7 in]
        n152 = call "Display Message to User"("error in (no error)"=w452) -> ("error out"=w442:errorcluster)  [unwired: 9 in, 1 out]
        n153 = Select(t=dbl[][] [[-8.43, -62.0, 4.0, 4.0], [-5.62, -59.0, 4.0, 4.0], [-2.81, -56.0, 4.0, 4.0], [0.0, -53.0, 1.0, 1.0], [-8.43, -48.0, 4.0, 0.0], [-5.62, -45.0, 4.0, 0.0], [-2.81, -42.0, 4.0, 0.0], [0.0, -39.0, 1.0, 0.0]], s=w416, f=dbl[][] [[-8.43, -48.0, 4.0, 4.0], [-5.62, -45.0, 4.0, 4.0], [-2.81, -42.0, 4.0, 4.0], [0.0, -39.0, 1.0, 1.0], [-8.43, -62.0, 4.0, 0.0], [-5.62, -59.0, 4.0, 0.0], [-2.81, -56.0, 4.0, 0.0], [0.0, -53.0, 1.0, 0.0]]) -> (s? t:f=w413:dbl[][])
        n154 = Index Array(array=w450, index=2) -> (element=w446:dbl)
        n155 = call-dynamic "Z Go.vi"("error in (no error)"=w442, "Speed"=20.0, "Position"=0.0, "Motion in"=w439) -> ("error out"=w438:errorcluster, "Motion out"=w445:refnum<class "Motion.lvclass">)  [unwired: 6 in]
        n156 = call "Display Message to User2"("error in (no error)"=w438) -> ("error out"=w437:errorcluster)  [unwired: 9 in, 1 out]
        n157 = Add(x=w446, y=-2.5) -> (x+y=w447:dbl)
        n158 = call-dynamic "Z Go.vi"("error in (no error)"=w437, "Speed"=20.0, "Position"=w447, "Motion in"=w445) -> ("error out"=w435:errorcluster, "Motion out"=w436:refnum<class "Motion.lvclass">)  [unwired: 6 in]
        n159 = call-dynamic "Connect.vi"("Ultimus V in"=refnum<class "Ultimus V2.lvclass"> refnum ("Ultimus V2.lvclass")) -> ("Ultimus V out"=w433:refnum<class "Ultimus V2.lvclass">)  [unwired: 9 in, 1 out]
        n160 = case shown="False" w425 {
          tunnel: w436 -> [w477 w580]
          tunnel: w435 -> [w478 w579]
          tunnel: [w476 w578] -> w430
          tunnel: [w478 w577] -> w428
          tunnel: w424 -> [w473 w571]
          tunnel: w434 -> [w472 w576]
          tunnel: w433 -> [w474 w575]
          tunnel: [w475 w574] -> w431
          tunnel: w423 -> [w471 w573]
          tunnel: w413 -> [w470 _]
          tunnel: "Needle Height Compenstation\n(glue gap)" -> [w469 w572]
          tunnel: "check height?" -> [w468 w569]
          tunnel: "Ultimus Pressure" -> [w467 w568]
          frame False {
            # "two sensor, Sensor B then A"
            n161 = for {
              N: w471 -> [_]
              tunnel: w477 -> [w495]
              tunnel: [w494] -> w475
              tunnel: [w493] -> w476
              tunnel: w474 -> [w492]
              tunnel: w473 -> [w491] mode=indexing
              tunnel: w472 -> [w485]
              tunnel: w470 -> [w487]
              tunnel: w469 -> [w481]
              tunnel: w468 -> [w480]
              tunnel: w467 -> [w479]
              i -> [w483]
              # "four\nloops"
              n162 = Multiply(x=4, y=w483) -> (x*y=w482:i32)
              n163 = Array Subset(array=w487, index (row)=w482, length (row)=4 ("length"), index (col)=0, length (col)=3 ("length")) -> (w486:dbl[][])
              "GlueBox" <- w486
              n164 = for {
                N: 4 -> [_]
                tunnel: w495 -> [w555]
                tunnel: [w547] -> w494
                tunnel: [w542] -> w493
                tunnel: w492 -> [w534]
                tunnel: w491 -> [w512]
                tunnel: w486 -> [w509] mode=indexing
                tunnel: w485 -> [w515]
                tunnel: w481 -> [w501]
                tunnel: w480 -> [w498]
                tunnel: w479 -> [w497]
                n165 = Index Array(array=w509, index=0) -> (element=w531:dbl)
                n166 = Index Array(array=w509, index=1) -> (element=w530:dbl)
                n167 = Array Subset(array=w512, index=0, length=2) -> (w514:dbl[])
                n168 = Add(x=w514, y=w515) -> (x+y=w513:dbl[])
                n169 = Absolute Value(x=w531) -> (abs(x)=w529:dbl)
                n170 = Absolute Value(x=w530) -> (abs(x)=w527:dbl)
                n171 = Add(x=w513, y=w509) -> (x+y=w524:dbl[])
                n172 = Multiply(x=w527, y=2.0) -> (x*y=w505:dbl)
                n173 = Multiply(x=w529, y=2.0) -> (x*y=w506:dbl)
                n174 = Multiply(x=w505, y=-1.0) -> (x*y=w517:dbl)
                n175 = Build Array(0.0 ("element"), w505) -> (w525:dbl[])
                n176 = Build Array(w506, 0.0 ("element")) -> (w522:dbl[])
                n177 = Build Array(0.0 ("element"), w517) -> (w503:dbl[])
                n178 = Add(x=w524, y=w525) -> (x+y=w521:dbl[])
                n179 = Add(x=w521, y=w522) -> (x+y=w504:dbl[])
                n180 = call-dynamic "XY Go.vi"("Speed"=200.0, "XY"=w524, "Motion in"=w555) -> ("error out"=w507:errorcluster, "Motion out"=w554:refnum<class "Motion.lvclass">)  [unwired: 7 in]
                n181 = Add(x=w504, y=w503) -> (x+y=w502:dbl[])
                n182 = Index Array(array=w512, index=2) -> (element=w511:dbl)
                n183 = Index Array(array=w509, index=2) -> (element=w508:dbl)
                n184 = Add(x=w511, y=w501) -> (x+y=w540:dbl)
                n185 = Build Array(w521, w504, w502, w524) -> (w516:dbl[][])
                "appended array" <- w516
                n186 = call-dynamic "Z Go.vi"("error in (no error)"=w507, "Speed"=5.0, "Position"=w540, "Motion in"=w554) -> ("error out"=w500:errorcluster, "Motion out"=w550:refnum<class "Motion.lvclass">)  [unwired: 6 in]
                n187 = case shown="True" w498 {
                  tunnel: w500 -> [w559 w561]
                  tunnel: [w559 w560] -> w499
                  frame False {
                  }
                  frame True {
                    n188 = call "Display Message to User11"("error in (no error)"=w561) -> ("error out"=w560:errorcluster)  [unwired: 9 in, 1 out]
                  }
                }
                n189 = call "vacuum.vi"("error in (no error)"=w499, "Vacuum Setting (0000)"=i64 100, "Ultimus V in"=w534) -> ("error out"=w552:errorcluster, "Ultimus V out"=w537:refnum<class "Ultimus V2.lvclass">)  [unwired: 7 in]
                n190 = call-dynamic "Pressure.vi"("error in (no error)"=w552, "Pressure"=w497, "Ultimus V in"=w537) -> ("error out"=w553:errorcluster, "Ultimus V out"=w536:refnum<class "Ultimus V2.lvclass">)  [unwired: 7 in]
                n191 = call-dynamic "Dispense.vi"("error in (no error)"=w553, "Ultimus V in"=w536) -> ("error out"=w549:errorcluster, "Ultimus V out"=w535:refnum<class "Ultimus V2.lvclass">)  [unwired: 8 in]
                n192 = for {
                  N: w508 -> [_]
                  tunnel: w550 -> [w567]
                  tunnel: w549 -> [w566]
                  tunnel: [w565] -> w548
                  tunnel: [w564] -> w546
                  tunnel: w516 -> [w563] mode=indexing
                  (unwired) 4.5 ("Speed")
                  n193 = call-dynamic "XY Go.vi"("error in (no error)"=w566, "Speed"=4.5, "XY"=w563, "Motion in"=w567) -> ("error out"=w565:errorcluster, "Motion out"=w564:refnum<class "Motion.lvclass">)  [unwired: 6 in]
                }
                n194 = Add(x=w540, y=-2.0) -> (x+y=w543:dbl)
                n195 = call-dynamic "Dispense.vi"("error in (no error)"=w548, "Ultimus V in"=w535) -> ("error out"=w541:errorcluster, "Ultimus V out"=w547:refnum<class "Ultimus V2.lvclass">)  [unwired: 8 in]
                n196 = call-dynamic "Z Go.vi"("error in (no error)"=w541, "Speed"=10.0, "Position"=w543, "Motion in"=w546) -> ("Motion out"=w542:refnum<class "Motion.lvclass">)  [unwired: 6 in, 1 out]
              }
            }
          }
          frame True {
            n197 = case shown="True" w569 {
              tunnel: w571 -> [w581 w585]
              tunnel: [w581 w582] -> w570
              frame False {
              }
              frame True {
                n198 = Array Subset(array=w585, index (row)=12 ("index"), length (row)=4 ("length")) -> (w582:dbl[][])  [unwired: 2 in]
              }
            }
            n199 = for {
              N: w573 -> [_]
              tunnel: w580 -> [w623]
              tunnel: w579 -> [w622]
              tunnel: [w608] -> w574
              tunnel: [w607] -> w578
              tunnel: [w606] -> w577
              tunnel: w570 -> [w594] mode=indexing
              tunnel: w576 -> [w593]
              tunnel: w575 -> [w592]
              tunnel: w572 -> [w590]
              tunnel: w569 -> [w587]
              tunnel: w568 -> [w586]
              # "move the glue in x-dir\n0.1 mm closer to center"
              n200 = Index Array(array=w594, index=2) -> (element=w595:dbl)
              n201 = Add(x=w594, y=w593) -> (x+y=w621:dbl[])
              n202 = Build Array(0.0 ("element"), 3.3 ("element")) -> (w626:dbl[])
              n203 = Subtract(x=w621, y=w626) -> (x-y=w627:dbl[])
              n204 = Add(x=w595, y=w590) -> (x+y=w596:dbl)
              n205 = Add(x=w621, y=w626) -> (x+y=w604:dbl[])
              n206 = call-dynamic "XY Go.vi"("error in (no error)"=w622, "Speed"=200.0, "XY"=w627, "Motion in"=w623) -> ("error out"=w609:errorcluster, "Motion out"=w602:refnum<class "Motion.lvclass">)  [unwired: 6 in]
              n207 = call-dynamic "Z Go.vi"("error in (no error)"=w609, "Speed"=5.0, "Position"=w596, "Motion in"=w602) -> ("error out"=w589:errorcluster)  [unwired: 6 in, 1 out]
              n208 = case shown="True" w587 {
                tunnel: w589 -> [w628 w630]
                tunnel: [w628 w629] -> w588
                frame False {
                }
                frame True {
                  n209 = call "Display Message to User7"("error in (no error)"=w630) -> ("error out"=w629:errorcluster)  [unwired: 9 in, 1 out]
                }
              }
              n210 = call "vacuum.vi"("error in (no error)"=w588, "Vacuum Setting (0000)"=i64 100, "Ultimus V in"=w592) -> ("error out"=w618:errorcluster, "Ultimus V out"=w613:refnum<class "Ultimus V2.lvclass">)  [unwired: 7 in]
              n211 = call-dynamic "Pressure.vi"("error in (no error)"=w618, "Pressure"=w586, "Ultimus V in"=w613) -> ("error out"=w619:errorcluster, "Ultimus V out"=w611:refnum<class "Ultimus V2.lvclass">)  [unwired: 7 in]
              n212 = call-dynamic "Dispense.vi"("error in (no error)"=w619, "Ultimus V in"=w611) -> ("error out"=w603:errorcluster, "Ultimus V out"=w610:refnum<class "Ultimus V2.lvclass">)  [unwired: 8 in]
              n213 = call "Time Delay"("error in (no error)"=w603) -> ("error out"=w601:errorcluster)  [unwired: 10 in]
              n214 = call-dynamic "XY Go.vi"("error in (no error)"=w601, "Speed"=5.0, "XY"=w604, "Motion in"=w602) -> ("error out"=w600:errorcluster, "Motion out"=w598:refnum<class "Motion.lvclass">)  [unwired: 6 in]
              n215 = call "Time Delay3"("error in (no error)"=w600) -> ("error out"=w599:errorcluster)  [unwired: 10 in]
              n216 = call "Time Delay2"("error in (no error)"=w601) -> ("error out"=w612:errorcluster)  [unwired: 10 in]
              n217 = call-dynamic "Dispense.vi"("error in (no error)"=w612, "Ultimus V in"=w610) -> ("Ultimus V out"=w608:refnum<class "Ultimus V2.lvclass">)  [unwired: 8 in, 1 out]
              n218 = Add(x=w596, y=-2.5) -> (x+y=w616:dbl)
              n219 = call-dynamic "Z Go.vi"("error in (no error)"=w599, "Speed"=10.0, "Position"=w616, "Motion in"=w598) -> ("error out"=w606:errorcluster, "Motion out"=w607:refnum<class "Motion.lvclass">)  [unwired: 6 in]
            }
          }
        }
        n220 = call-dynamic "Disconnect.vi"("Ultimus V in"=w431) -> ()  [unwired: 9 in, 1 out]
        n221 = call "XYZTheta Go.vi"("error in (no error)"=w428, "XYZTheta In"=dbl[] [800.0, 800.0, 0.0, 0.1], "Motion in"=w430) -> ("error out"=w429:errorcluster, "Motion out"=w426:refnum<class "Motion.lvclass">)  [unwired: 6 in, 1 out]
        n222 = call "Display Message to User3"("error in (no error)"=w429) -> ()  [unwired: 9 in, 2 out]
      }
      event "Needle Alignment": Value Change {
        (unwired) "Needle Alignment in progress ...." ("String")
        # "first needle park position\nneedle gap on Z value : 0.5 mm"
        # "Syringe-camera offset"
        n223 = event-data() -> ()  [unwired: 1 in, 6 out]
        n224 = call-poly <vilib>:"Read Delimited Spreadsheet.vi"("file path (dialog if empty)"=path "D:/INTT/V1/Assembly Data/Tool Offsets/Dispense Tip Offset.txt", "number of rows (all:-1)"=-1) -> ("first row"=w672:dbl[])  [unwired: 8 in, 5 out]
        n225 = Build Array(11.75, -25, 0.5 ("element"), 0.0 ("element")) -> (w665:dbl[])
        n226 = Index Array(array=w672, index #1=0 ("index"), index #2=1 ("index")) -> (element #1=w667:dbl, element #2=w664:dbl)
        n227 = Build Array(w667, w664, 0.0 ("element"), 0.0 ("element")) -> (w634:dbl[])
        n228 = Add(x=w634, y=w665) -> (x+y=w658:dbl[])
        n229 = Add(x=w657, y=w658) -> (x+y=w659:dbl[])
        n230 = call "XYZTheta Go.vi"("XYZTheta In"=w659, "Motion in"=w649) -> ("error out"=w663:errorcluster, "XYZTheta Out"=w639:dbl[], "Motion out"=w648:refnum<class "Motion.lvclass">)  [unwired: 7 in]
        n231 = call "Display Message to User10"("error in (no error)"=w663) -> ("error out"=w660:errorcluster)  [unwired: 9 in, 1 out]
        n232 = call-dynamic "Z Go.vi"("error in (no error)"=w660, "Speed"=20.0, "Position"=0.0, "Motion in"=w648) -> ("Motion out"=w647:refnum<class "Motion.lvclass">)  [unwired: 6 in, 1 out]
        n233 = Replace Array Subset(array=w639, new element=0.0 ("new element/subarray"), index=2) -> (w636:dbl[])
        n234 = call "Joystick and Camera - external Connection.vi"("Motion in"=w647, "XYZTheta"=w636, "Measurement Point"="Touch Needle on a surface") -> ("Motion out"=w645:refnum<class "Motion.lvclass">, "Gantry"=w635:dbl[])  [unwired: 4 in, 2 out]
        n235 = Subtract(x=w635, y=w634) -> (x-y=w633:dbl[])
        n236 = call "Joystick and Camera - external Connection.vi"("Motion in"=w645, "XYZTheta"=w633, "Measurement Point"="Measure the touch spot with camera") -> ("Motion out"=w641:refnum<class "Motion.lvclass">, "Gantry"=w644:dbl[])  [unwired: 4 in, 2 out]
        n237 = Subtract(x=w635, y=w644) -> (x-y=w643:dbl[])
        n238 = call-poly <vilib>:"Write Delimited Spreadsheet.vi"("file path (dialog if empty)"=path "D:/INTT/V1/Assembly Data/Tool Offsets/Dispense Tip Offset.txt", "1D data"=w643, "append to file? (new file:F)"=FALSE) -> ()  [unwired: 11 in, 2 out]
      }
      event "Pick and place": Value Change {
        (unwired) "PICK and PLACE samples ..." ("String")
        (unwired) -21.3804 ("new element/subarray")
        n239 = event-data() -> ()  [unwired: 1 in, 6 out]
        n240 = call-poly <vilib>:"Read Delimited Spreadsheet.vi"("file path (dialog if empty)"=path "D:/INTT/V1/Assembly Data/Tool Offsets/Bellows Tool Offset.txt", "number of rows (all:-1)"=-1) -> ("first row"=w702:dbl[])  [unwired: 8 in, 5 out]
        n241 = Select(t=1, s=w679, f=w691) -> (s? t:f=w707:i32)
        n242 = Index Array(array=w702, index #1=0 ("index"), index #2=1 ("index"), index #3=2 ("index")) -> (element #1=w698:dbl, element #2=w697:dbl, element #3=w696:dbl)
        n243 = case shown="True" w687 {
          tunnel: [w708 w711] -> w686
          tunnel: w681 -> [w708 w710]
          frame False {
          }
          frame True {
            # "sensor A"
            # "sensor B"
            n244 = Index Array(array=w710, index=0) -> (element=w709:i32)
            n245 = Index Array(array=w710, index=1) -> (element=w712:i32)
            n246 = Build Array(w712, w709) -> (w711:i32[])
          }
        }
        n247 = for {
          N: w707 -> [_]
          tunnel: w691 -> [w751]
          tunnel: w692 -> [w747]
          tunnel: w705 -> [w771]
          tunnel: [w759] -> w695
          tunnel: w693 -> [w769] mode=indexing
          tunnel: [w735] -> w685
          tunnel: w684 -> [w722]
          tunnel: w698 -> [w761]
          tunnel: w697 -> [w760]
          tunnel: w694 -> [w744]
          tunnel: w696 -> [w758]
          tunnel: w679 -> [w728]
          tunnel: w686 -> [w716] mode=indexing
          tunnel: "VacChannel for sample" -> [w730]
          tunnel: "check height? 2" -> [w723]
          tunnel: w679 -> [w715]
          i -> [w737]
          w720 = 0 ("Channel")
          w719 = TRUE ("Value")
          # "put back pickup tool"
          # "if chips, do one pickup tool and multiple samples;\nif sensors, one pickup tool for one sample ( so 2->2);"
          # "build a fake 2d arrays"
          # "sensor"
          # "chip pickup tool"
          # "pickup tool height offset"
          # "Pick up PICKUP TOOL"
          # "Pick up CHIPs/Sensor and place on HDI"
          n248 = Select(t=w751, s=w728, f=1) -> (s? t:f=w750:i32)
          n249 = Build Array(w761, w760, w758, 0.0 ("element")) -> (w756:dbl[])
          n250 = Add(x=w769, y=w756) -> (x+y=w757:dbl[])
          n251 = call "XYZTheta-2Zspeed Go.vi"("XYZTheta In"=w757, "Motion in"=w771) -> ("error out"=w718:errorcluster, "Motion out"=w770:refnum<class "Motion.lvclass">)  [unwired: 7 in, 1 out]
          n252 = Select(t=-18.52 ("new element/subarray"), s=w728, f=-13.13 ("t")) -> (s? t:f=w752:dbl)
          n253 = call "WriteReadWait.vi"("Read Value"=w719, "Write Value"=w719, "error in (no error)"=w718, "Read"=w720, "Write"=w720, "I-O in"=w722) -> ("error out"=w717:errorcluster, "I-O out"=w721:refnum<class "NI-DAQ.lvclass">)  [unwired: 4 in]
          n254 = Replace Array Subset(array=w756, new element=w752, index=2) -> (w754:dbl[])
          n255 = Index Array(array=w747, index (row)=w737) -> (element=w746:dbl[])  [unwired: 1 in]
          n256 = call "Time Delay8"("error in (no error)"=w717) -> ("error out"=w767:errorcluster)  [unwired: 10 in]
          n257 = Build Array(w746, w746) -> (w745:dbl[][])
          n258 = Select(t=w747, s=w728, f=w745) -> (s? t:f=w748:dbl[][])
          n259 = Index Array(array=w744, index (row)=w737) -> (element=w743:dbl[])  [unwired: 1 in]
          n260 = Build Array(w743, w743) -> (w742:dbl[][])
          n261 = Select(t=w744, s=w728, f=w742) -> (s? t:f=w725:dbl[][])
          n262 = case shown="True" w723 {
            tunnel: [w772 w774] -> w724
            tunnel: w725 -> [w772 w773]
            frame False {
            }
            frame True {
              n263 = Array Subset(array=w773, index (row)=12 ("index"), length (row)=4 ("length")) -> (w774:dbl[][])  [unwired: 2 in]
            }
          }
          n264 = Select(t="chip placement height compensation", s=w728, f=0.0) -> (s? t:f=w726:dbl)
          n265 = for {
            N: w750 -> [_]
            tunnel: w748 -> [w791] mode=indexing
            tunnel: w770 -> [w793]
            tunnel: w754 -> [w792]
            tunnel: w767 -> [w790]
            tunnel: [w789] -> w762
            tunnel: w721 -> [w788]
            tunnel: w724 -> [w785] mode=indexing
            tunnel: [w784] -> w753
            tunnel: w726 -> [w783]
            tunnel: w716 -> [w782]
            tunnel: w730 -> [w781]
            tunnel: [w780] -> w729
            tunnel: w728 -> [w779]
            tunnel: w723 -> [w778]
            tunnel: w715 -> [w777]
            n266 = flat-sequence {
              tunnel: w791 -> [w810]
              tunnel: [w812] -> w794
              tunnel: w793 -> [w811]
              tunnel: w792 -> [w809]
              tunnel: w790 -> [w807]
              tunnel: w788 -> [w805]
              tunnel: [w799] -> w787
              tunnel: [w800] -> w786
              tunnel: w782 -> [w802]
              tunnel: w781 -> [w797]
              tunnel: w794 -> [w835]
              tunnel: [w834] -> w789
              tunnel: w792 -> [w832]
              tunnel: w787 -> [w833]
              tunnel: w786 -> [w820]
              tunnel: w785 -> [w831]
              tunnel: [w814] -> w784
              tunnel: w783 -> [w824]
              tunnel: w781 -> [w819]
              tunnel: [w815] -> w780
              tunnel: w779 -> [_]
              tunnel: w778 -> [w821]
              tunnel: w777 -> [w813]
              frame #0 {
                w798 = TRUE ("Value")
                w801 = FALSE ("Value")
                # "pickup sample"
                # "release sample from tray"
                # "pickup sample from tray"
                n267 = Add(x=w810, y=w809) -> (x+y=w808:dbl[])
                n268 = call "XYZTheta-2Zspeed Go.vi"("error in (no error)"=w807, "XYZTheta In"=w808, "Motion in"=w811) -> ("error out"=w806:errorcluster, "Motion out"=w812:refnum<class "Motion.lvclass">)  [unwired: 6 in, 1 out]
                n269 = call "Time Delay4"("error in (no error)"=w806) -> ("error out"=w803:errorcluster)  [unwired: 10 in]
                n270 = call "WriteReadWait.vi"("Read Value"=w801, "Write Value"=w801, "error in (no error)"=w803, "Read"=w802, "Write"=w802, "I-O in"=w805) -> ("error out"=w804:errorcluster, "I-O out"=w796:refnum<class "NI-DAQ.lvclass">)  [unwired: 4 in]
                n271 = call "Time Delay11"("error in (no error)"=w804) -> ("error out"=w795:errorcluster)  [unwired: 10 in]
                n272 = call "WriteReadWait.vi"("Read Value"=w798, "Write Value"=w798, "error in (no error)"=w795, "Read"=w797, "Write"=w797, "I-O in"=w796) -> ("error out"=w799:errorcluster, "I-O out"=w800:refnum<class "NI-DAQ.lvclass">)  [unwired: 4 in]
              }
              frame #1 {
                w817 = FALSE ("Value")
                # "release sample on HDI"
                # "lift for chip/sensor thickness"
                # "place sample on HDI"
                n273 = Add(x=w831, y=w832) -> (x+y=w827:dbl[])
                n274 = Build Array(0.0 ("element"), 0.0 ("element"), w824, 0.0 ("element")) -> (w826:dbl[])
                n275 = Add(x=w827, y=w826) -> (x+y=w825:dbl[])
                n276 = call "XYZTheta-2Zspeed Go.vi"("error in (no error)"=w833, "XYZTheta In"=w825, "Motion in"=w835) -> ("error out"=w823:errorcluster, "Motion out"=w834:refnum<class "Motion.lvclass">)  [unwired: 6 in, 1 out]
                n277 = case shown="True" w821 {
                  tunnel: w823 -> [w840 w842]
                  tunnel: [w840 w841] -> w822
                  frame False {
                  }
                  frame True {
                    n278 = call "Display Message to User6"("error in (no error)"=w842) -> ("error out"=w841:errorcluster)  [unwired: 9 in, 1 out]
                  }
                }
                n279 = case shown="True" w813 {
                  tunnel: w822 -> [w837 w839]
                  tunnel: [w836 w838] -> w818
                  frame False {
                    n280 = call "Time Delay7"("error in (no error)"=w837) -> ("error out"=w836:errorcluster)  [unwired: 10 in]
                  }
                  frame True {
                    n281 = call "Time Delay6"("error in (no error)"=w839) -> ("error out"=w838:errorcluster)  [unwired: 10 in]
                  }
                }
                n282 = call "WriteReadWait.vi"("Read Value"=w817, "Write Value"=w817, "error in (no error)"=w818, "Read"=w819, "Write"=w819, "I-O in"=w820) -> ("error out"=w816:errorcluster, "I-O out"=w815:refnum<class "NI-DAQ.lvclass">)  [unwired: 4 in]
                n283 = call "Time Delay5"("error in (no error)"=w816) -> ("error out"=w814:errorcluster)  [unwired: 10 in]
              }
            }
          }
          n284 = call "XYZTheta-2Zspeed Go.vi"("error in (no error)"=w753, "XYZTheta In"=w757, "Motion in"=w762) -> ("error out"=w727:errorcluster, "Motion out"=w766:refnum<class "Motion.lvclass">)  [unwired: 6 in, 1 out]
          n285 = call "Time Delay9"("error in (no error)"=w727) -> ("error out"=w733:errorcluster)  [unwired: 10 in]
          n286 = call-dynamic "Digital Write 1 Channel.vi"("DAQ Module"=0, "error constant"=w733, "Value"=FALSE, "Channel"=0, "NI-DAQ.lvclass"=w729) -> ("error IO"=w736:errorcluster, "NI-DAQ.lvclass 2"=w735:refnum<class "NI-DAQ.lvclass">)  [unwired: 5 in]
          n287 = call "Time Delay10"("error in (no error)"=w736) -> ("error out"=w763:errorcluster)  [unwired: 10 in]
          n288 = call-dynamic "Z Go.vi"("error in (no error)"=w763, "Speed"=20.0, "Position"=0.0 ("new element/subarray"), "Motion in"=w766) -> ("Motion out"=w759:refnum<class "Motion.lvclass">)  [unwired: 6 in, 1 out]
        }
      }
      event "GOTO": Value Change {
        (unwired) "GOING to a position" ("String")
        n289 = event-data() -> ()  [unwired: 1 in, 6 out]
        n290 = call "XYZTheta-2Zspeed Go.vi"("XYZTheta In"="Parking position", "Motion in"=w846) -> ("Motion out"=w845:refnum<class "Motion.lvclass">)  [unwired: 7 in, 2 out]
      }
      event "READ Position": Value Change {
        n291 = event-data() -> ()  [unwired: 1 in, 6 out]
        n292 = call-dynamic "Get Current Position.vi"("Motion in"=w868) -> ("XYZTheta Out"=→"Gantry current position":dbl[], "Motion out"=w867:refnum<class "Motion.lvclass">)  [unwired: 8 in, 1 out]
      }
      event "TrayVaccum": Value Change {
        n293 = event-data() -> ()  [unwired: 1 in, 6 out]
        n294 = Index Array(array=w871, index=0) -> (element=w880:i32)
        n295 = Index Array(array="Values", index=0) -> (element=w874:bool)
        n296 = call "WriteReadWait.vi"("Read Value"=w874, "Write Value"=w874, "Read"=w880, "Write"=w880, "I-O in"=w883) -> ("error out"=w879:errorcluster, "I-O out"=w882:refnum<class "NI-DAQ.lvclass">)  [unwired: 5 in]
        n297 = Index Array(array=w871, index=1) -> (element=w877:i32)
        n298 = Index Array(array="Values", index=1) -> (element=w872:bool)
        n299 = call "WriteReadWait.vi"("Read Value"=w872, "Write Value"=w872, "error in (no error)"=w879, "Read"=w877, "Write"=w877, "I-O in"=w882) -> ("I-O out"=w869:refnum<class "NI-DAQ.lvclass">)  [unwired: 4 in, 1 out]
      }
      event Timeout {
        n300 = event-data() -> ()  [unwired: 1 in, 3 out]
        n301 = call-dynamic "Digital Read Multiple Channels.vi"("Array"=w896, "NI-DAQ in"=w895) -> ("subarray"=w897:bool[], "NI-DAQ out"=w893:refnum<class "NI-DAQ.lvclass">)  [unwired: 7 in, 1 out]
      }
    }
    "Measure HDI top-left" <- w36
    "Sample on HDI" <- w14
    "vacuum on?" <- w10
    n302 = feedback-in #1(w34) -> ()
    n303 = feedback-in #2(w36) -> ()
    n304 = feedback-in #3(w31) -> ()
    n305 = feedback-in #4(w23) -> ()
    n306 = feedback-in #5(w20) -> ()
    n307 = feedback-in #6(w10) -> ()
    n308 = feedback-in #7(w28) -> ()
    n309 = feedback-in #8(w14) -> ()
    n310 = feedback-in #9(w29) -> ()
    "# of tasks excuted" <- w25
  }
  n311 = call-dynamic "Disconnect.vi"("I-O in"=w1) -> ()  [unwired: 9 in, 1 out]
  n312 = call-dynamic "Disconnect.vi"("Controller in"=w4) -> ()  [unwired: 9 in, 1 out]
